vi "Main.vi"() -> ()   [LabVIEW 2014]
uses:
  Types/Lamp.ctl
  Types/TempCont.ctl
  Types/HeatingMode.ctl
  Types/Cases.ctl
  Types/DataCluster.ctl
  Types/Humans.ctl
  Types/HumanArray.ctl
  Types/Rooms.ctl
  Types/TemperatureControlData.ctl
  Types/RoomPositions.ctl
  <vilib>/Utility/miscctls.llb/LVPositionTypeDef.ctl
  Types/StartingPositions.ctl
  Types/LightCases.ctl
  Types/TemperatureArray.ctl
  Types/FVGFuncts.ctl
  <vilib>/Utility/error.llb/DialogType.ctl
  Types/MoveActions.ctl
  <vilib>/Utility/error.llb/Error Cluster From Error Code.vi
  <vilib>/Utility/file.llb/Read From Spreadsheet File (string).vi
  <vilib>/ErrorRing/Error Ring.xnode
panel:
  in  "Update Settings":bool
  out "F0 Temp Chart":dbl(graph)
  out "F1 Temp Chart":dbl(graph)
  out "Kinti hõmérséklet":dbl
  out "F1 Gain":dbl
  out "F0 Gain":dbl
  out "RIASZTÁS":bool
  out "Óra":string
  in  "Nyitott ablakok":i8 min=0 max=13 step=1
  in  "Riasztó":bool
  out "Vezérlés F1":T1
  out "Fûtési hõm. F1":dbl
  out "Aktuális hõm. F1":dbl
  in  "Kívánt hõm. F1":T2=22.0 min=10.0 max=30.0 step=0.5
  out "Vezérlés F0":T1
  out "Fûtési hõm. F0":dbl
  out "Aktuális hõm. F0":dbl
  in  "Kívánt hõm. F0":T2=22.0 min=10.0 max=30.0 step=0.5
  in  "Világítás":bool
  out "Stopped":bool
  out "EM Lámpa":T3
  out "LH Lámpa":T3
  out "EF Lámpa":T3
  out "HSZ1 Lámpa":T3
  out "HSZ2 Lámpa":T3
  out "KÉ Lámpa":T3
  out "FM Lámpa":T3
  out "FF Lámpa":T3
  out "N Lámpa":T3
  out "B Lámpa":T3
  in  "Choose Button":bool
  in  "Human 6 Button":bool
  in  "Human 5 Button":bool
  in  "Human 4 Button":bool
  in  "Human 3 Button":bool
  in  "Human 2 Button":bool
  in  "Human 1 Button":bool
  in  "Remove Button":bool
  in  "Add Button":bool
  in  "Next Button":bool
  in  "Previous Button":bool
  in  "Down Button":bool
  in  "Up Button":bool
  in  "Stop Button":bool
  in  "Human 6":u16(ring)
  in  "Human 5":u16(ring)
  in  "Human 4":u16(ring)
  in  "Human 3":u16(ring)
  in  "Human 2":u16(ring)
  in  "Human 1":u16(ring)
  # "Családtagok"
  # "Navigáció"
  # "Elsõ Emeleti Termosztát"
  # "Földszinti Termosztát"
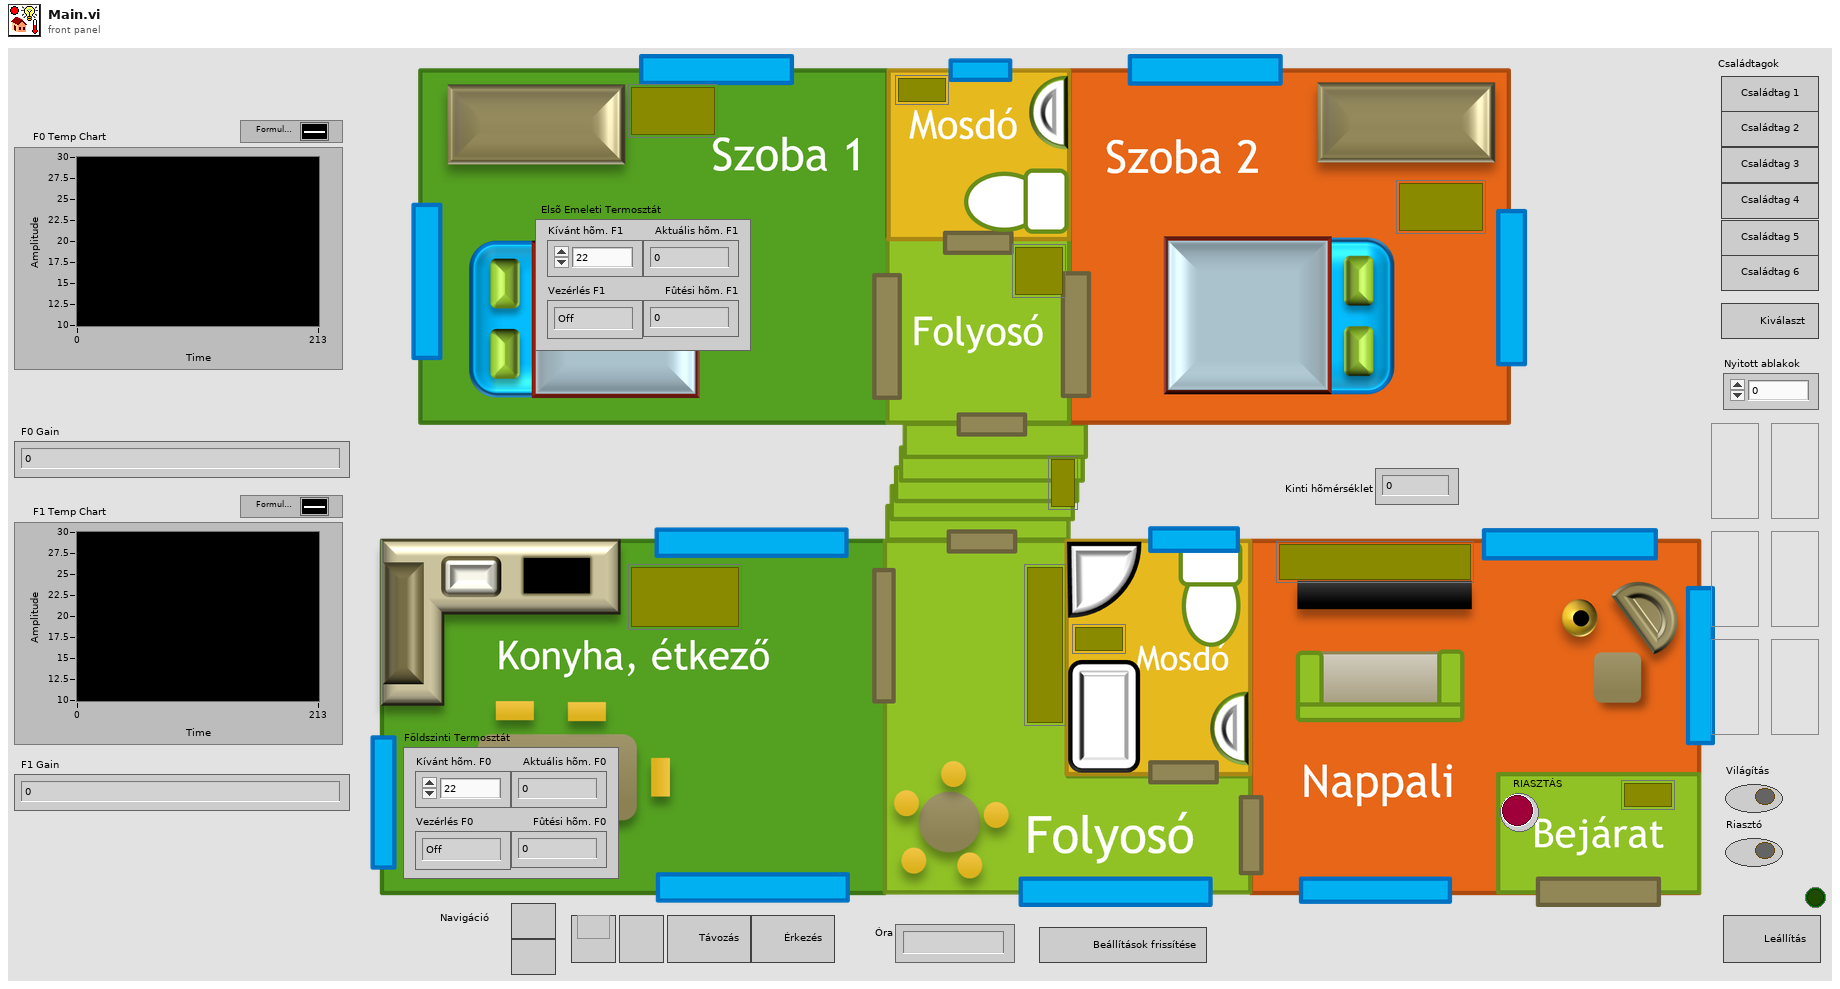
[diagram p1: front panel]
types:
  T1 = typedef "HeatingMode.ctl" = enum16{"Off", "Heating", "Cooling"}
  T2 = typedef "TempCont.ctl" = dbl
  T3 = typedef "Lamp.ctl" = bool
  T4 = typedef "LightCases.ctl" = enum16{"Start", "Update", "Stop"}
  T5 = typedef "FVGFuncts.ctl" = enum16{"Init", "Set Data", "Get Data"}
  T6 = typedef "TemperatureArray.ctl" = dbl[]
  T7 = typedef "TemperatureControlData.ctl" = cluster{"Open windows":dbl, "Floor 0 Heating":T1, "Floor 1 Heating":T1, "Heating Temp":dbl}
  T8 = typedef "HumanArray.ctl" = T9[]
  T9 = typedef "Rooms.ctl" = enum16{"Sehol", "Elõszoba", "Nappali", "Konyha", "Földszinti mosdó", "Földszinti folyosó", "Lépcsõ", "Emeleti folyosó", "Emeleti mosdó", "Hálószoba 1", "Hálószoba 2"}
  T10 = typedef "StartingPositions.ctl" = T11[]
  T11 = typedef "LVPositionTypeDef.ctl" = cluster{"Left":i32, "Top":i32}
  T12 = typedef "RoomPositions.ctl" = T11[]
  T13 = typedef "DataCluster.ctl" = cluster{"Controlled Human":T14, "Human Positions":T8, "NumOfHumans":u8, "TemperatureData":T7, "Floor0 Temp":dbl, "Floor1 Temp":dbl}
  T14 = typedef "Humans.ctl" = enum16{"No Human", "Human 1", "Human 2", "Human 3", "Human 4", "Human 5", "Human 6"}
  T15 = typedef "Cases.ctl" = enum16{"Init", "UpdateWord", "UpdateHuman", "UpdatePositions", "UpdateHeating", "UpdateTemperature", "UpdateLights", "Close", "Stop"}
  T16 = typedef "MoveActions.ctl" = enum16{"Move", "Get in", "Leave"}
  T17 = typedef "DialogType.ctl" = u16
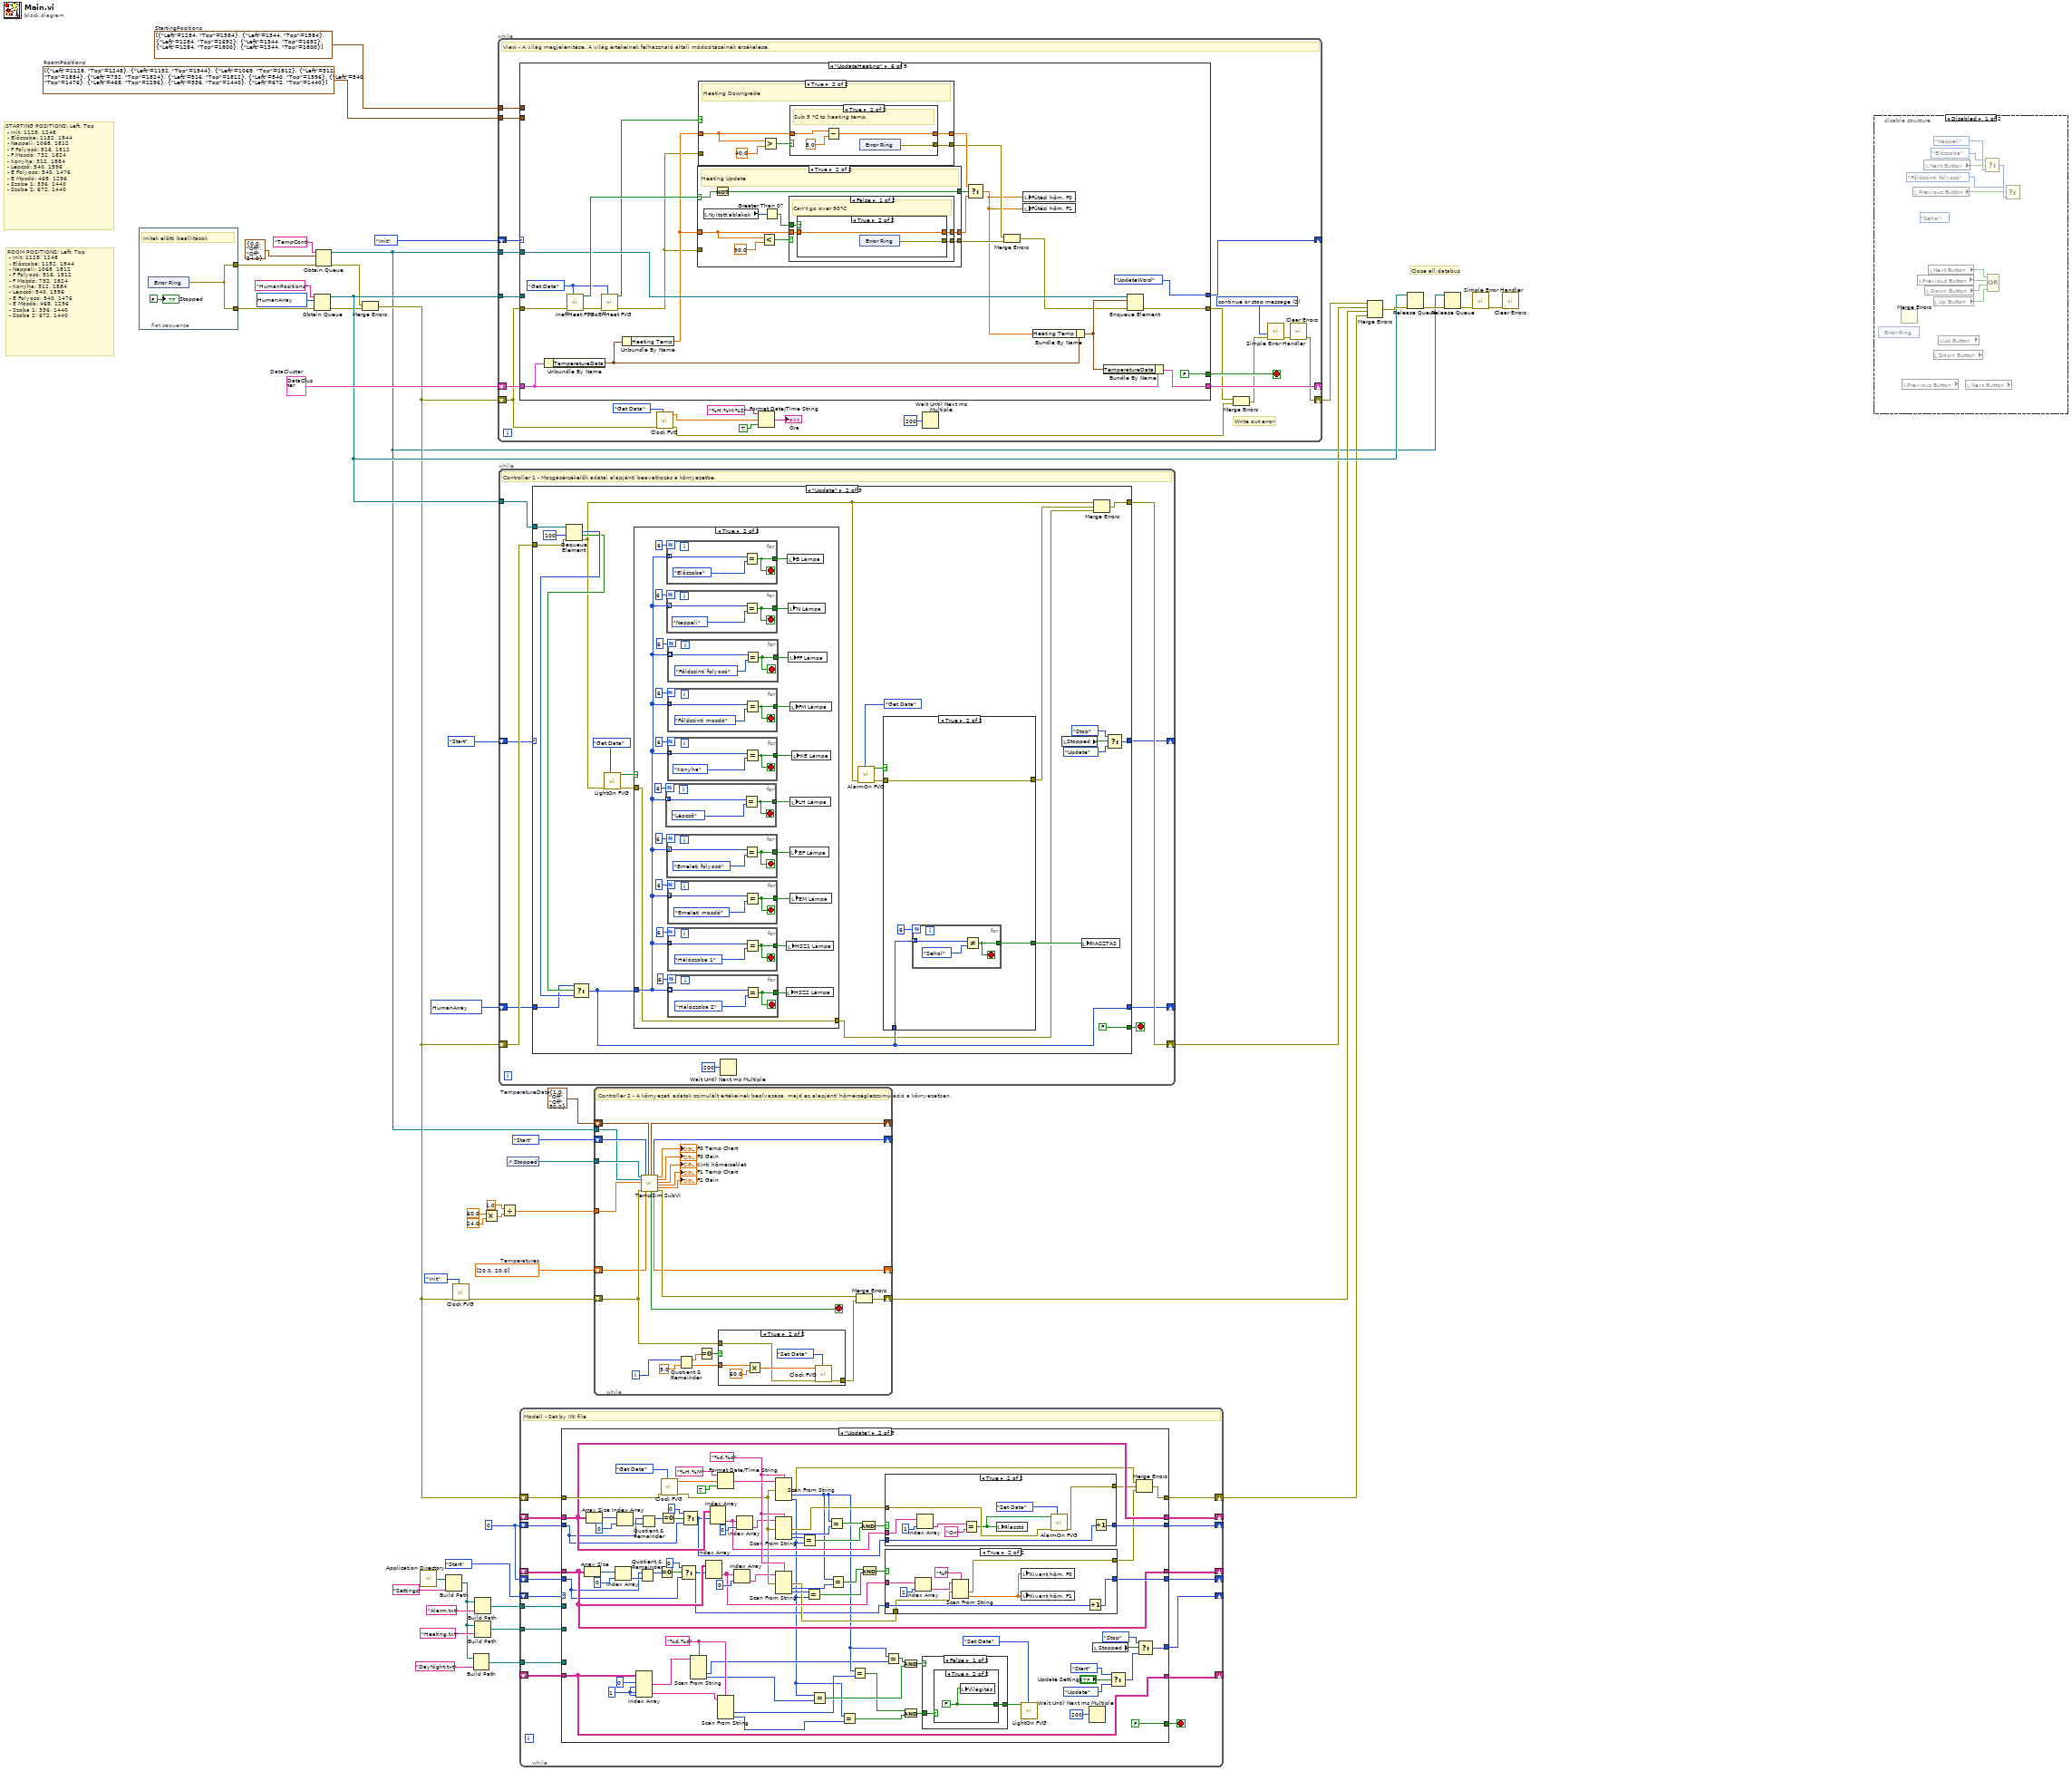
[diagram p0: block diagram]
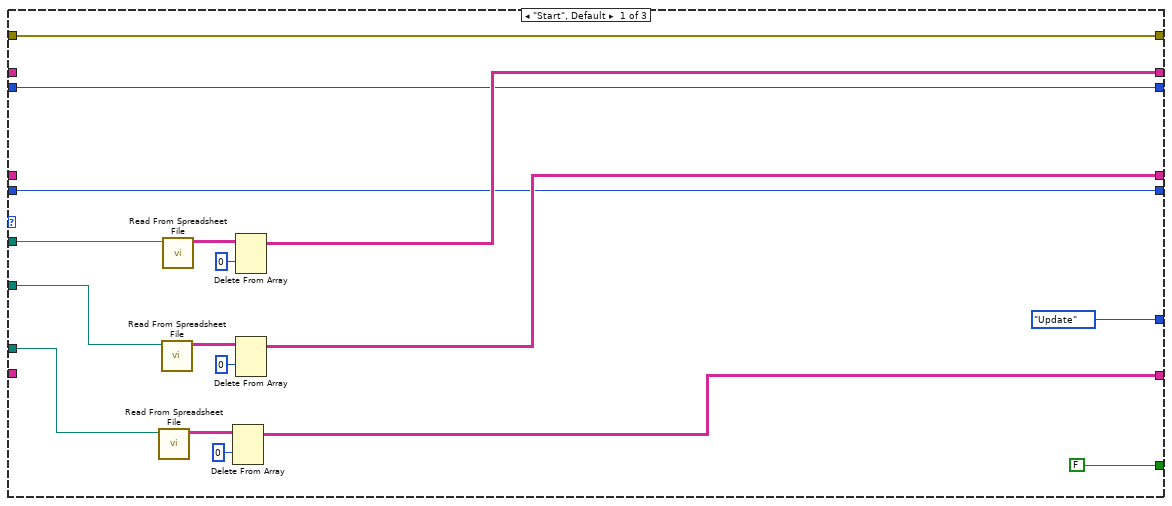
[diagram p2: hidden frame]
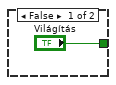
[diagram p3: hidden frame]
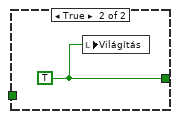
[diagram p4: hidden frame]
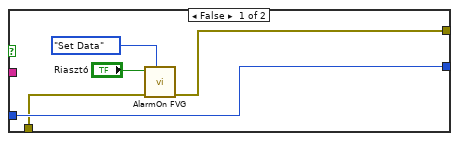
[diagram p5: hidden frame]
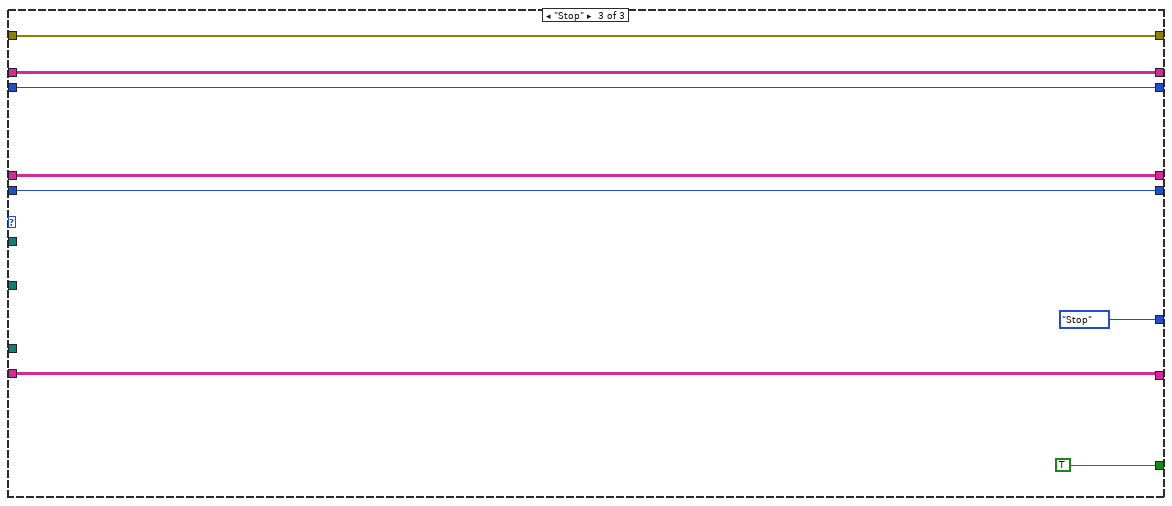
[diagram p7: hidden frame]
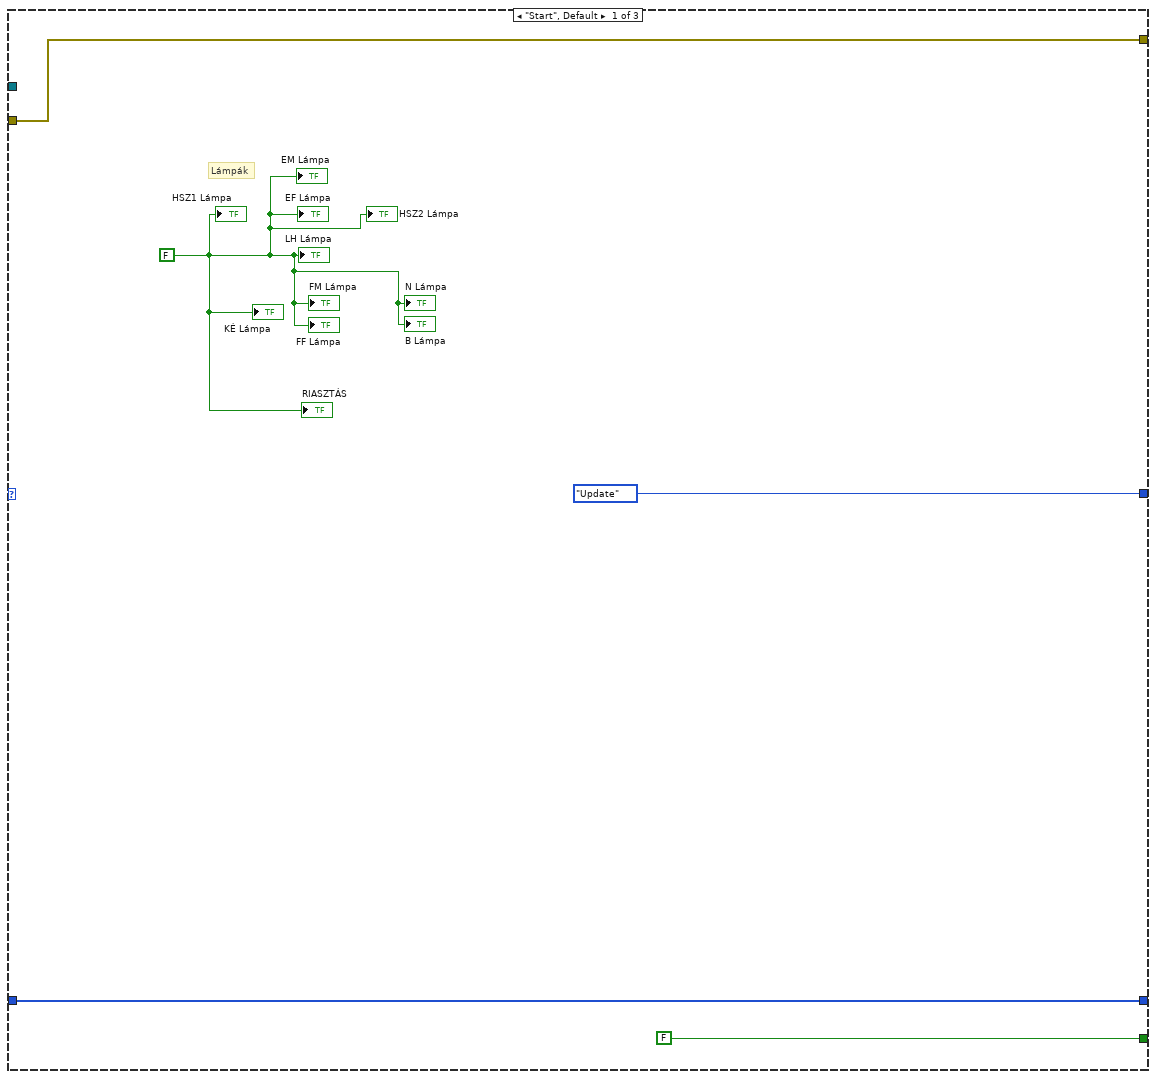
[diagram p9: hidden frame]
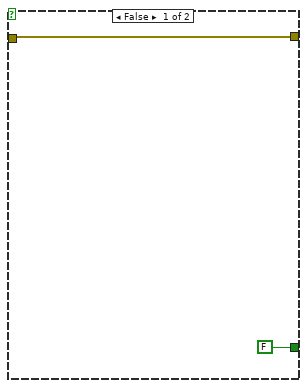
[diagram p10: hidden frame]
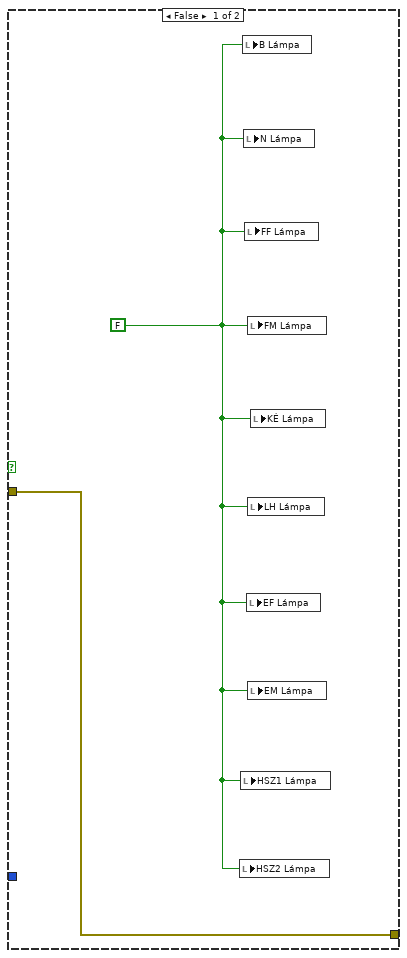
[diagram p11: hidden frame]
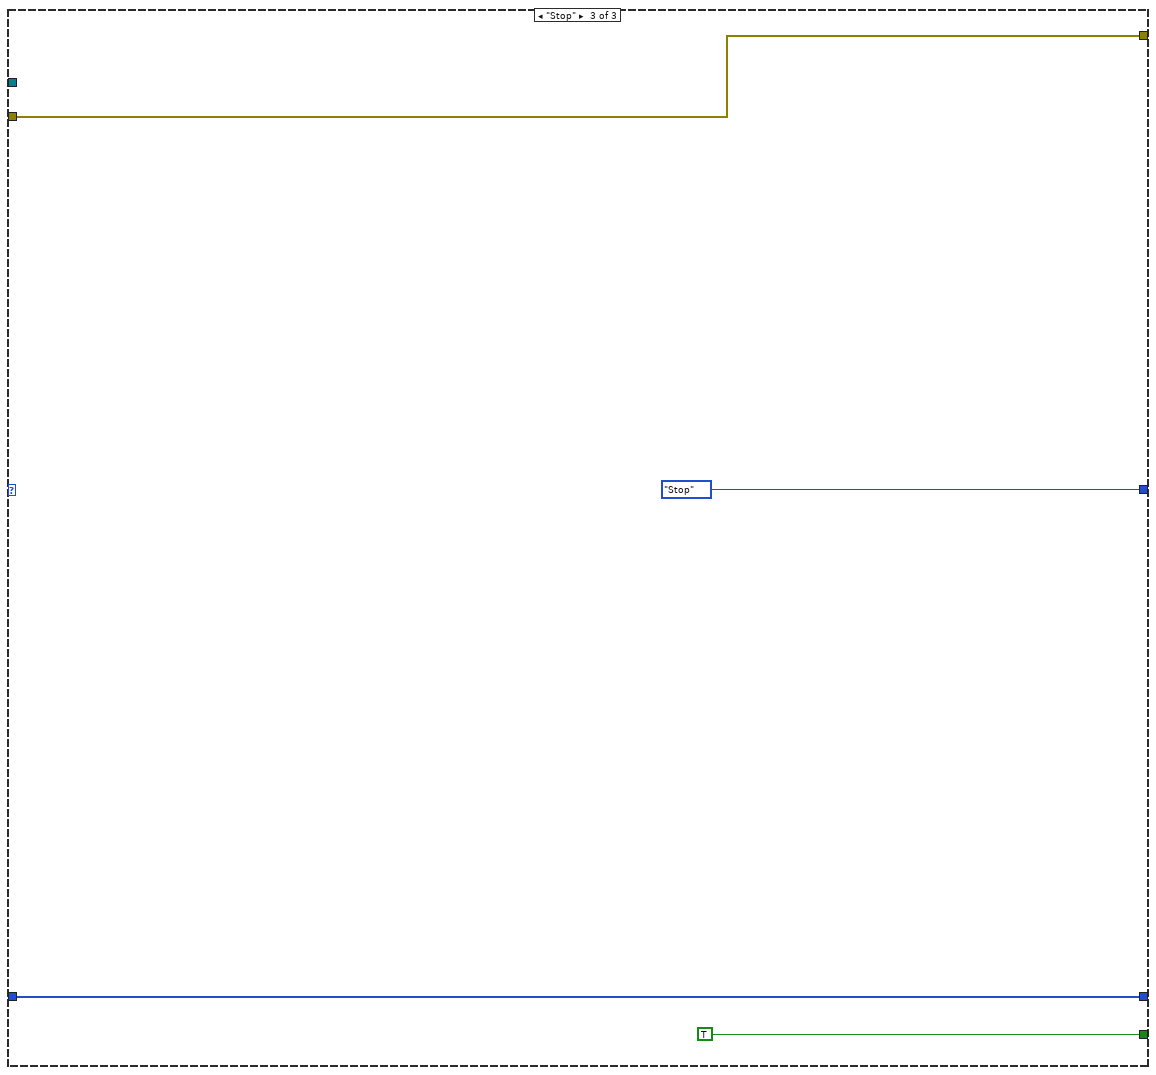
[diagram p12: hidden frame]
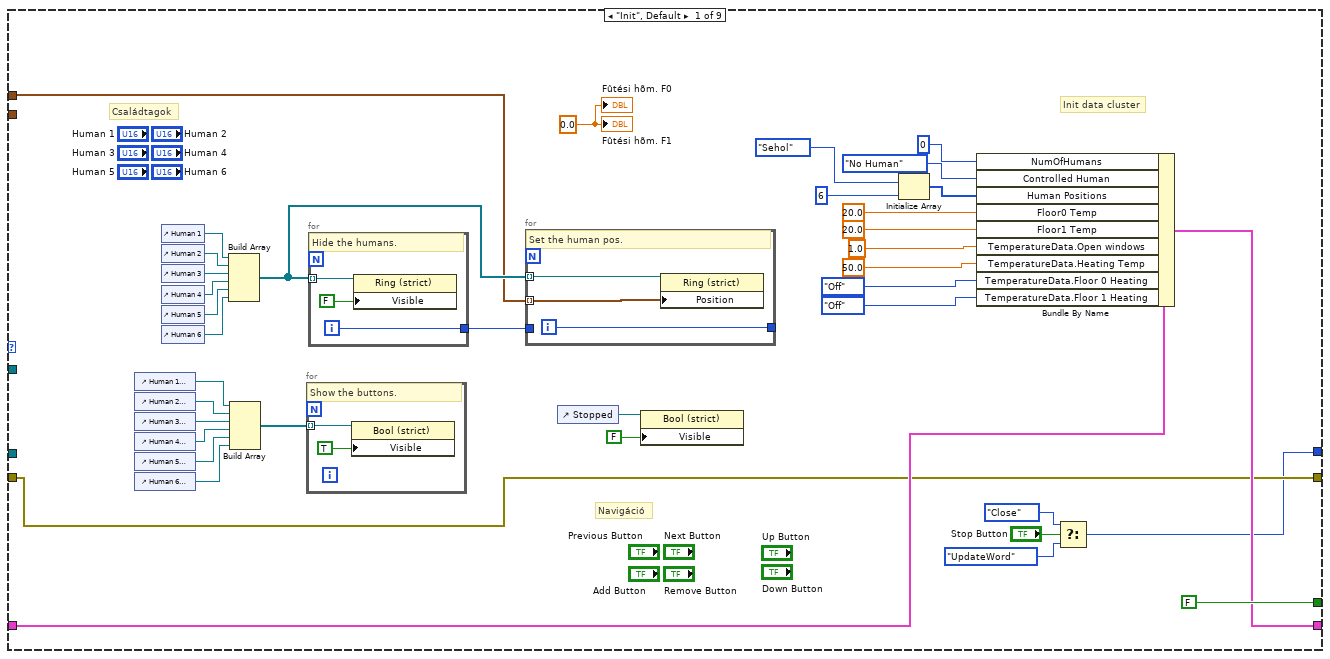
[diagram p14: hidden frame]
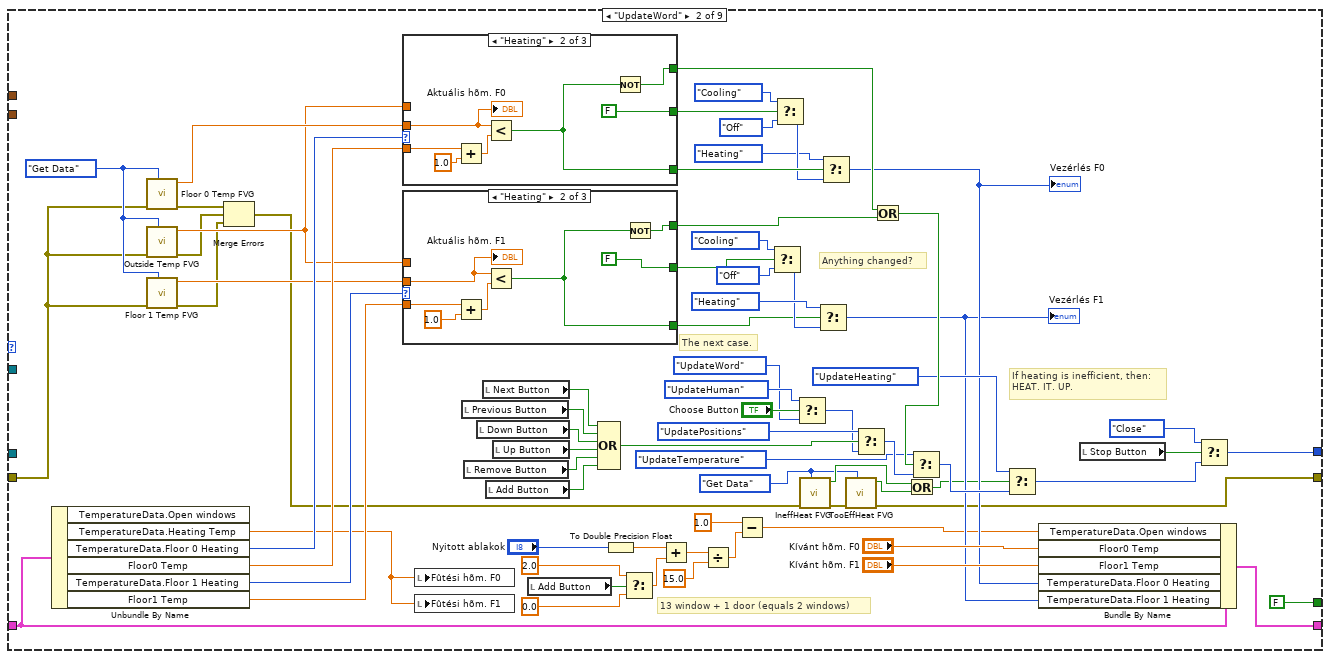
[diagram p15: hidden frame]
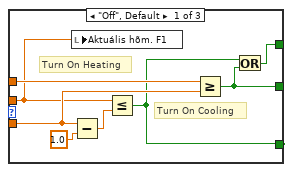
[diagram p16: hidden frame]
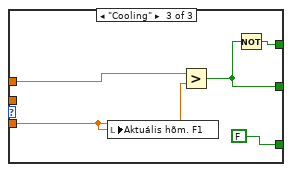
[diagram p17: hidden frame]
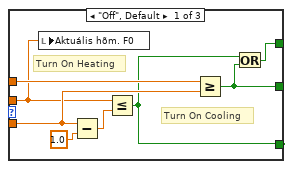
[diagram p18: hidden frame]
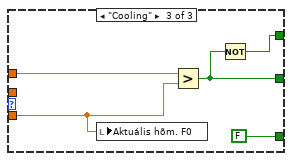
[diagram p19: hidden frame]
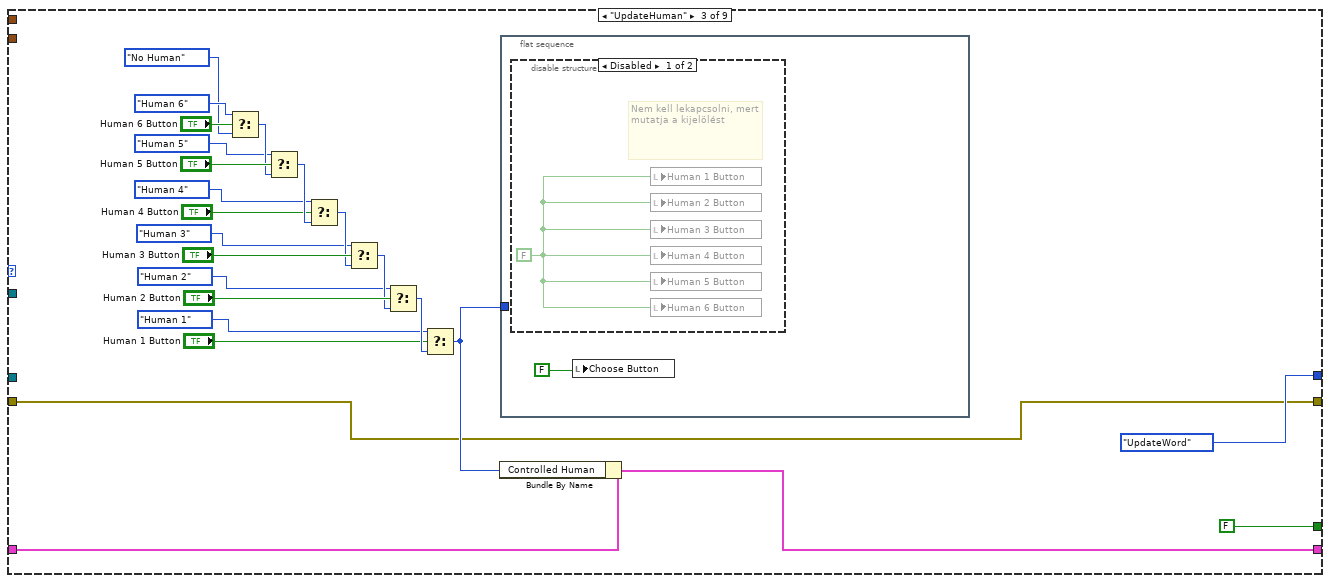
[diagram p20: hidden frame]
diagram:
  w3 = 0 ("index (row)")
  w21 = T6 [20.0, 20.0]  # Temperatures
  w22 = T7 {"Open windows"=1.0, "Floor 0 Heating"=enum."Off", "Floor 1 Heating"=enum."Off", "Heating Temp"=50.0}  # TemperatureData
  w36 = T8 [enum."Sehol", enum."Sehol", enum."Sehol", enum."Sehol", enum."Sehol", enum."Sehol", enum."Sehol", enum."Sehol", enum."Sehol", enum."Sehol", enum."Sehol", enum."Sehol"] items=["Sehol", "Elõszoba", "Nappali", "Konyha", "Földszinti mosdó", "Földszinti folyosó", "Lépcsõ", "Emeleti folyosó", "Emeleti mosdó", "Hálószoba 1", "Hálószoba 2"] ("Human Positions")
  w43 = T8 [enum."Sehol", enum."Sehol", enum."Sehol", enum."Sehol", enum."Sehol", enum."Sehol", enum."Sehol", enum."Sehol", enum."Sehol", enum."Sehol", enum."Sehol", enum."Sehol"] items=["Sehol", "Elõszoba", "Nappali", "Konyha", "Földszinti mosdó", "Földszinti folyosó", "Lépcsõ", "Emeleti folyosó", "Emeleti mosdó", "Hálószoba 1", "Hálószoba 2"] ("Human Positions")
  w44 = T10 [{"Left"=1284, "Top"=1584}, {"Left"=1344, "Top"=1584}, {"Left"=1284, "Top"=1692}, {"Left"=1344, "Top"=1692}, {"Left"=1284, "Top"=1800}, {"Left"=1344, "Top"=1800}]  # StartingPositions
  w45 = T12 [{"Left"=1128, "Top"=1248}, {"Left"=1152, "Top"=1944}, {"Left"=1068, "Top"=1812}, {"Left"=312, "Top"=1884}, {"Left"=732, "Top"=1824}, {"Left"=516, "Top"=1812}, {"Left"=540, "Top"=1596}, {"Left"=540, "Top"=1476}, {"Left"=468, "Top"=1296}, {"Left"=336, "Top"=1440}, {"Left"=672, "Top"=1440}]  # RoomPositions
  w46 = T13 {"Controlled Human"=enum."No Human", "Human Positions"=[], "NumOfHumans"=0, "TemperatureData"={"Open windows"=1.0, "Floor 0 Heating"=enum."Off", "Floor 1 Heating"=enum."Off", "Heating Temp"=50.0}, "Floor0 Temp"=24.0, "Floor1 Temp"=24.0}  # DataCluster
  # "Close all databus"
  # "STARTING POSITIONS: Left, Top\n - Init: 1128, 1248 \n - Elõszoba: 1152, 1944\n - Nappali: 1068, 1812\n - F Folyosó: 516, 1812\n - F Mosdó: 732, 1824 \n - Konyha: 312, 1884\n - Lépcsõ: 540, 1596\n - E Folyosó: 540, 1476\n - E Mosdó: 468, 1296\n - Szoba 1: 336, 1440\n - Szoba 2: 672, 1440"
  # "ROOM POSITIONS: Left, Top\n - Init: 1128, 1248 \n - Elõszoba: 1152, 1944\n - Nappali: 1068, 1812\n - F Folyosó: 516, 1812\n - F Mosdó: 732, 1824 \n - Konyha: 312, 1884\n - Lépcsõ: 540, 1596\n - E Folyosó: 540, 1476\n - E Mosdó: 468, 1296\n - Szoba 1: 336, 1440\n - Szoba 2: 672, 1440"
  n1 = flat-sequence {
    tunnel: [w48] -> w41
    tunnel: [w48] -> w35
    frame #0 {
      # "Initek elõtti beállítások"
      n2 = xnode "Error Ring"() -> ("error out"=w48:errorcluster)
      "Stopped" <- FALSE ("Stopped")
    }
  }
  n3 = Obtain Queue(name (unnamed)="HumanPositions", element data type=w43, error in (no error)=w41) -> (queue out=w39:refnum<queue>, error out=w31:errorcluster)  [unwired: 2 in, 1 out]
  n4 = Obtain Queue(name (unnamed)="TempCont", element data type=T7 {"Open windows"=0.0, "Floor 0 Heating"=enum."Off", "Floor 1 Heating"=enum."Off", "Heating Temp"=24.0} ("TemperatureData"), error in (no error)=w35) -> (queue out=w7:refnum<queue>, error out=w32:errorcluster)  [unwired: 2 in, 1 out]
  n5 = Merge Errors(w32, w31) -> (w15:errorcluster)
  n6 = call <vilib>:"Application Directory.vi"() -> ("Application Directory"=w13:path)
  n7 = Build Path(base path=w13, name or relative path="Settings") -> (appended path=w4:path)
  n8 = call "Clock FVG.vi"("Mode"=FVGFuncts."Init" ("Enum"), "Error In"=w15) -> ("Error Out"=w20:errorcluster)  [unwired: 8 in, 1 out]
  n9 = Build Path(base path=w4, name or relative path="DayNight.txt") -> (appended path=w5:path)
  n10 = Build Path(base path=w4, name or relative path="Alarm.txt") -> (appended path=w9:path)
  n11 = Build Path(base path=w4, name or relative path="Heating.txt") -> (appended path=w8:path)
  n12 = Multiply(x=60.0, y=24.0) -> (x*y=w29:dbl)
  n13 = while {
    shift-right: [w65] -> _
    shift-left: Cases."Init" -> [w72]
    shift-right: [w69] -> _
    shift-left: w46 -> [w70]
    tunnel: w45 -> [w64]
    tunnel: w44 -> [w63]
    tunnel: w39 -> [w67]
    shift-right: [w51] -> w24
    shift-left: w15 -> [w55]
    tunnel: w7 -> [w66]
    stop <- w71 stop-if-true
    w53 = T17 2 items=["no dialog", "OK message", "continue or stop message", "OK message + warnings", "continue/stop + warnings"] ("type of dialog (OK msg:1)")
    # "Write out error"
    # "View - A világ megjelenítése, A világ értékeinek felhasználó általi módositásainak érzékelése."
    n14 = case shown="\"UpdateHeating\"" w72 {
      tunnel: [FALSE FALSE FALSE FALSE FALSE FALSE FALSE FALSE TRUE] -> w71
      tunnel: [w74 w136 Cases."UpdateWord" Cases."UpdateLights" Cases."UpdateWord" Cases."UpdateWord" Cases."UpdateWord" Cases."Stop" Cases."Stop"] -> w65
      tunnel: w70 -> [w109 w154 w235 w268 w480 w501 w557 w579 w590]
      tunnel: [w105 w153 w234 w263 w480 w500 w557 w579 w590] -> w69
      tunnel: w64 -> [_ _ _ w264 _ _ _ _ _]
      tunnel: w63 -> [w88 _ _ _ _ _ _ _ _]
      tunnel: w55 -> [w86 w174 w232 w259 w478 w503 w560 w564 w589]
      tunnel: w67 -> [_ _ _ _ w479 _ _ _ _]
      tunnel: [w86 w121 w232 w258 w476 w499 w559 w564 w589] -> w59
      tunnel: w66 -> [_ _ _ _ _ w496 w558 _ _]
      frame "Init", Default {
        w73 = 0.0 ("Fûtési hõm. F1")
        # "Családtagok"
        # "Navigáció"
        # "Init data cluster"
        n15 = control-ref of="Human 1 Button"() -> (w92:refnum<vi>)
        n16 = control-ref of="Human 2 Button"() -> (w91:refnum<vi>)
        n17 = control-ref of="Human 3 Button"() -> (w96:refnum<vi>)
        n18 = control-ref of="Human 4 Button"() -> (w93:refnum<vi>)
        n19 = control-ref of="Human 5 Button"() -> (w94:refnum<vi>)
        n20 = control-ref of="Human 6 Button"() -> (w95:refnum<vi>)
        n21 = control-ref of="Human 1"() -> (w101:refnum<vi>)
        n22 = control-ref of="Human 2"() -> (w100:refnum<vi>)
        n23 = control-ref of="Human 3"() -> (w102:refnum<vi>)
        n24 = control-ref of="Human 4"() -> (w97:refnum<vi>)
        n25 = control-ref of="Human 5"() -> (w98:refnum<vi>)
        n26 = control-ref of="Human 6"() -> (w99:refnum<vi>)
        n27 = Build Array(w101, w100, w102, w97, w98, w99) -> (w89:refnum<vi>[])
        n28 = Build Array(w92, w91, w96, w93, w94, w95) -> (w90:refnum<vi>[])
        n29 = for {
          tunnel: w90 -> [w115] mode=indexing
          # "Show the buttons."
          n30 = property class="Bool (strict)"(reference=w115, "Visible"=TRUE) -> ()  [unwired: 1 in, 2 out]
        }
        n31 = for {
          tunnel: [w118] -> w87
          tunnel: w89 -> [w117] mode=indexing
          i -> [w118]
          # "Hide the humans."
          n32 = property class="Ring (strict)"(reference=w117, "Visible"=FALSE) -> ()  [unwired: 1 in, 2 out]
        }
        n33 = for {
          tunnel: [w113] -> _
          tunnel: w89 -> [w112] mode=indexing
          tunnel: w88 -> [w111] mode=indexing
          tunnel: w87 -> [_]
          i -> [w113]
          # "Set the human pos."
          n34 = property class="Ring (strict)"(reference=w112, "Position"=w111) -> ()  [unwired: 1 in, 2 out]
        }
        n35 = control-ref of="Stopped"() -> (w84:refnum<vi>)
        n36 = property class="Bool (strict)"(reference=w84, "Visible"=FALSE) -> ()  [unwired: 1 in, 2 out]
        n37 = Initialize Array(Rooms."Sehol" ("element"), 6 ("dimension size")) -> (w106:T9[])
        n38 = Bundle By Name(cluster=w109, "NumOfHumans"=u8 0, "Controlled Human"=Humans."No Human", "Human Positions"=w106, "Floor0 Temp"=20.0 ("Floor 0 Temperature"), "Floor1 Temp"=20.0 ("Floor 0 Temperature"), "TemperatureData.Open windows"=1.0 ("Floor 0 Temperature"), "TemperatureData.Heating Temp"=50.0 ("Floor 0 Temperature"), "TemperatureData.Floor 0 Heating"=HeatingMode."Off" ("Floor 0 Heating"), "TemperatureData.Floor 1 Heating"=HeatingMode."Off" ("Floor 0 Heating")) -> (w105:T13)
        n39 = Select(t=Cases."Close", s="Stop Button", f=Cases."UpdateWord") -> (s? t:f=w74:T15)
        "Fûtési hõm. F1" <- w73
        "Fûtési hõm. F0" <- w73
      }
      frame "UpdateWord" {
        w123 = FVGFuncts."Get Data" ("Mode")
        w175 = FVGFuncts."Get Data" ("Enum")
        # "13 window + 1 door (equals 2 windows)"
        # "If heating is inefficient, then: \nHEAT. IT. UP."
        # "Anything changed?"
        # "The next case."
        n40 = Unbundle By Name(w154) -> ("TemperatureData.Heating Temp"=w142:dbl, "TemperatureData.Floor 0 Heating"=w176:T1, "Floor0 Temp"=w177:dbl, "TemperatureData.Floor 1 Heating"=w172:T1, "Floor1 Temp"=w173:dbl)  [unwired: 1 out]
        n41 = call "Floor 0 Temp FVG.vi"("Mode"=w175, "Error In"=w174) -> ("Error Out"=w157:errorcluster, "Data Out"=w178:dbl)  [unwired: 8 in]
        n42 = call "Outside Temp FVG.vi"("Mode"=w175, "Error In"=w174) -> ("Error Out"=w155:errorcluster, "Data Out"=w170:dbl)  [unwired: 8 in]
        n43 = call "Floor 1 Temp FVG.vi"("Mode"=w175, "Error In"=w174) -> ("Error Out"=w156:errorcluster, "Data Out"=w171:dbl)  [unwired: 8 in]
        n44 = Merge Errors(w157, w155, w156) -> (w140:errorcluster)
        n45 = case shown="\"Heating\"" w176 {
          tunnel: w178 -> [w212 w220 _]
          tunnel: w177 -> [w217 w226 w227]
          tunnel: w170 -> [w216 _ w230]
          tunnel: [w214 w221 FALSE] -> w168
          tunnel: [w215 FALSE w229] -> w169
          tunnel: [w213 w222 w228] -> w149
          frame "Off", Default {
            # "Turn On Cooling"
            # "Turn On Heating"
            n46 = local write "Aktuális hõm. F0"(w212) -> ()
            n47 = Subtract(x=w217, y=1.0) -> (x-y=w218:dbl)
            n48 = Less Or Equal?(x=w212, y=w218) -> (x <= y?=w214:bool)
            n49 = Greater Or Equal?(x=w216, y=w217) -> (x >= y?=w215:bool)
            n50 = Or(x=w214, y=w215) -> (x .or. y?=w213:bool)
          }
          frame "Heating" {
            n51 = Add(x=w226, y=1.0) -> (x+y=w224:dbl)
            n52 = Less?(x=w220, y=w224) -> (x < y?=w221:bool)
            n53 = Not(x=w221) -> (.not. x?=w222:bool)
            "Aktuális hõm. F0" <- w220
          }
          frame "Cooling" {
            n54 = local write "Aktuális hõm. F0"(w227) -> ()
            n55 = Greater?(x=w230, y=w227) -> (0:w229:bool)
            n56 = Not(x=w229) -> (.not. x?=w228:bool)
          }
        }
        n57 = case shown="\"Heating\"" w172 {
          tunnel: w171 -> [w192 w200 _]
          tunnel: w173 -> [w197 w206 w207]
          tunnel: w170 -> [w196 _ w210]
          tunnel: [w194 w201 FALSE] -> w159
          tunnel: [w193 FALSE w209] -> w158
          tunnel: [w195 w202 w208] -> w150
          frame "Off", Default {
            # "Turn On Cooling"
            # "Turn On Heating"
            n58 = local write "Aktuális hõm. F1"(w192) -> ()
            n59 = Subtract(x=w197, y=1.0) -> (x-y=w198:dbl)
            n60 = Less Or Equal?(x=w192, y=w198) -> (x <= y?=w194:bool)
            n61 = Greater Or Equal?(x=w196, y=w197) -> (x >= y?=w193:bool)
            n62 = Or(x=w194, y=w193) -> (x .or. y?=w195:bool)
          }
          frame "Heating" {
            n63 = Add(x=w206, y=1.0) -> (x+y=w204:dbl)
            n64 = Less?(x=w200, y=w204) -> (x < y?=w201:bool)
            n65 = Not(x=w201) -> (.not. x?=w202:bool)
            "Aktuális hõm. F1" <- w200
          }
          frame "Cooling" {
            n66 = local write "Aktuális hõm. F1"(w207) -> ()
            n67 = Greater?(x=w210, y=w207) -> (0:w209:bool)
            n68 = Not(x=w209) -> (.not. x?=w208:bool)
          }
        }
        n69 = local write "Fûtési hõm. F0"(w142) -> ()
        n70 = local write "Fûtési hõm. F1"(w142) -> ()
        n71 = local read "Previous Button"() -> (w182:bool)
        n72 = local read "Remove Button"() -> (w183:bool)
        n73 = local read "Down Button"() -> (w186:bool)
        n74 = local read "Next Button"() -> (w185:bool)
        n75 = local read "Add Button"() -> (w184:bool)
        n76 = local read "Up Button"() -> (w187:bool)
        n77 = local read "Add Button"() -> (w128:bool)
        n78 = Compound Arithmetic op=OR(w185, w182, w186, w187, w183, w184) -> (w180:bool)
        n79 = To Double Precision Float(number="Nyitott ablakok") -> (double precision float=w132:dbl)
        n80 = Select(t=2.0, s=w128, f=0.0) -> (s? t:f=w131:dbl)
        n81 = Add(x=w132, y=w131) -> (x+y=w127:dbl)
        n82 = Divide(x=w127, y=15.0) -> (x/y=w125:dbl)
        n83 = Subtract(x=1.0, y=w125) -> (x-y=w135:dbl)
        n84 = Select(t=HeatingMode."Cooling" ("HeatingMode"), s=w158, f=HeatingMode."Off" ("HeatingMode")) -> (s? t:f=w160:T1)
        n85 = Select(t=HeatingMode."Cooling" ("HeatingMode"), s=w169, f=HeatingMode."Off" ("HeatingMode")) -> (s? t:f=w167:T1)
        n86 = Select(t=Cases."UpdateHuman", s="Choose Button", f=Cases."UpdateWord") -> (s? t:f=w141:T15)
        n87 = call "IneffHeat FVG.vi"("Mode"=w123, "Error In"=w140) -> ("Error Out"=w122:errorcluster, "Data Out"=w124:bool)  [unwired: 8 in]
        n88 = Select(t=HeatingMode."Heating" ("HeatingMode"), s=w159, f=w160) -> (s? t:f=w143:T1)
        "Vezérlés F1" <- w143
        n89 = Select(t=HeatingMode."Heating" ("HeatingMode"), s=w168, f=w167) -> (s? t:f=w144:T1)
        "Vezérlés F0" <- w144
        n90 = call "TooEffHeat FVG.vi"("Mode"=w123, "Error In"=w122) -> ("Error Out"=w121:errorcluster, "Data Out"=w120:bool)  [unwired: 8 in]
        n91 = Select(t=Cases."UpdatePositions", s=w180, f=w141) -> (s? t:f=w179:T15)
        n92 = Or(x=w149, y=w150) -> (x .or. y?=w148:bool)
        n93 = Or(x=w124, y=w120) -> (x .or. y?=w119:bool)
        n94 = Select(t=Cases."UpdateTemperature", s=w148, f=w179) -> (s? t:f=w146:T15)
        n95 = Select(t=Cases."UpdateHeating", s=w119, f=w146) -> (s? t:f=w137:T15)
        n96 = Bundle By Name(cluster=w154, "TemperatureData.Open windows"=w135, "Floor0 Temp"="Kívánt hõm. F0", "Floor1 Temp"="Kívánt hõm. F1", "TemperatureData.Floor 0 Heating"=w144, "TemperatureData.Floor 1 Heating"=w143) -> (w153:T13)
        n97 = local read "Stop Button"() -> (w139:bool)
        n98 = Select(t=Cases."Close", s=w139, f=w137) -> (s? t:f=w136:T15)
      }
      frame "UpdateHuman" {
        n99 = Select(t=Humans."Human 6", s="Human 6 Button", f=Humans."No Human") -> (s? t:f=w251:T14)
        n100 = Select(t=Humans."Human 5", s="Human 5 Button", f=w251) -> (s? t:f=w248:T14)
        n101 = Select(t=Humans."Human 4", s="Human 4 Button", f=w248) -> (s? t:f=w245:T14)
        n102 = Select(t=Humans."Human 3", s="Human 3 Button", f=w245) -> (s? t:f=w243:T14)
        n103 = Select(t=Humans."Human 2", s="Human 2 Button", f=w243) -> (s? t:f=w242:T14)
        n104 = Select(t=Humans."Human 1", s="Human 1 Button", f=w242) -> (s? t:f=w233:T14)
        n105 = Bundle By Name(cluster=w235, "Controlled Human"=w233) -> (w234:T13)
        n106 = flat-sequence {
          tunnel: w233 -> [_]
          frame #0 {
            n107 = disable-structure shown="Disabled" {
              frame Disabled {
                w257 = FALSE
                # "Nem kell lekapcsolni, mert mutatja a kijelölést"
                n108 = local write "Human 1 Button"(w257) -> ()
                n109 = local write "Human 2 Button"(w257) -> ()
                n110 = local write "Human 3 Button"(w257) -> ()
                n111 = local write "Human 4 Button"(w257) -> ()
                n112 = local write "Human 5 Button"(w257) -> ()
                n113 = local write "Human 6 Button"(w257) -> ()
              }
              frame Enabled {
              }
            }
            n114 = local write "Choose Button"(FALSE) -> ()
          }
        }
      }
      frame "UpdatePositions" {
        # "Choose the moving type. \n(Works if only 1 can be true)"
        n115 = local read "Remove Button"() -> (w272:bool)
        n116 = local read "Add Button"() -> (w271:bool)
        n117 = Unbundle By Name(w268) -> ("Human Positions"=w274:T8, "Controlled Human"=w276:T14, "NumOfHumans"=w265:u8)
        n118 = Select(t=MoveActions."Get in", s=w271, f=MoveActions."Move") -> (s? t:f=w261:T16)
        n119 = Select(t=MoveActions."Leave", s=w272, f=w261) -> (s? t:f=w269:T16)
        n120 = case shown="\"Get in\"" w269 {
          tunnel: w276 -> [w287 w383 w430]
          tunnel: w274 -> [w283 w386 w440]
          tunnel: [w282 w385 w438] -> w267
          tunnel: [w281 w392 w431] -> w266
          tunnel: w265 -> [w281 w393 w432]
          tunnel: w264 -> [w280 w384 w439]
          tunnel: [w279 w391 w437] -> w258
          tunnel: w259 -> [w278 w381 w428]
          frame "Move", Default {
            # "Who moves?"
            # "Where it can move?"
            n121 = Decrement(x=w287) -> (x-1=w284:T14)
            n122 = Index Array(array=w283, index=w284) -> (element=w286:T9)
            n123 = case shown="\"Sehol\", Default" w286 {
              tunnel: [Rooms."Sehol" ("element") w291 w295 w302 w306 w310 w323 w330 w343 w347 w351] -> w285
              frame "Sehol", Default {
              }
              frame "Elõszoba" {
                n124 = local read "Previous Button"() -> (w294:bool)
                n125 = Select(t=Rooms."Nappali" ("element"), s=w294, f=Rooms."Elõszoba" ("element")) -> (s? t:f=w291:T9)
              }
              frame "Nappali" {
                n126 = local read "Previous Button"() -> (w299:bool)
                n127 = local read "Next Button"() -> (w301:bool)
                n128 = Select(t=Rooms."Elõszoba" ("element"), s=w301, f=Rooms."Nappali" ("element")) -> (s? t:f=w296:T9)
                n129 = Select(t=Rooms."Földszinti folyosó" ("element"), s=w299, f=w296) -> (s? t:f=w295:T9)
              }
              frame "Konyha" {
                n130 = local read "Next Button"() -> (w305:bool)
                n131 = Select(t=Rooms."Földszinti folyosó" ("element"), s=w305, f=Rooms."Konyha" ("element")) -> (s? t:f=w302:T9)
              }
              frame "Földszinti mosdó" {
                n132 = local read "Down Button"() -> (w309:bool)
                n133 = Select(t=Rooms."Földszinti folyosó" ("element"), s=w309, f=Rooms."Földszinti mosdó" ("element")) -> (s? t:f=w306:T9)
              }
              frame "Földszinti folyosó" {
                n134 = local read "Previous Button"() -> (w320:bool)
                n135 = local read "Down Button"() -> (w319:bool)
                n136 = local read "Next Button"() -> (w322:bool)
                n137 = local read "Up Button"() -> (w318:bool)
                n138 = Select(t=Rooms."Nappali" ("element"), s=w322, f=Rooms."Földszinti folyosó" ("element")) -> (s? t:f=w317:T9)
                n139 = Select(t=Rooms."Konyha" ("element"), s=w320, f=w317) -> (s? t:f=w315:T9)
                n140 = Select(t=Rooms."Földszinti mosdó" ("element"), s=w319, f=w315) -> (s? t:f=w312:T9)
                n141 = Select(t=Rooms."Lépcsõ" ("element"), s=w318, f=w312) -> (s? t:f=w310:T9)
              }
              frame "Lépcsõ" {
                n142 = local read "Down Button"() -> (w327:bool)
                n143 = local read "Up Button"() -> (w329:bool)
                n144 = Select(t=Rooms."Emeleti folyosó" ("element"), s=w329, f=Rooms."Lépcsõ" ("element")) -> (s? t:f=w324:T9)
                n145 = Select(t=Rooms."Földszinti folyosó" ("element"), s=w327, f=w324) -> (s? t:f=w323:T9)
              }
              frame "Emeleti folyosó" {
                n146 = local read "Previous Button"() -> (w340:bool)
                n147 = local read "Down Button"() -> (w339:bool)
                n148 = local read "Next Button"() -> (w342:bool)
                n149 = local read "Up Button"() -> (w338:bool)
                n150 = Select(t=Rooms."Hálószoba 2" ("element"), s=w342, f=Rooms."Emeleti folyosó" ("element")) -> (s? t:f=w337:T9)
                n151 = Select(t=Rooms."Hálószoba 1" ("element"), s=w340, f=w337) -> (s? t:f=w335:T9)
                n152 = Select(t=Rooms."Lépcsõ" ("element"), s=w339, f=w335) -> (s? t:f=w332:T9)
                n153 = Select(t=Rooms."Emeleti mosdó" ("element"), s=w338, f=w332) -> (s? t:f=w330:T9)
              }
              frame "Emeleti mosdó" {
                n154 = local read "Down Button"() -> (w346:bool)
                n155 = Select(t=Rooms."Emeleti folyosó" ("element"), s=w346, f=Rooms."Emeleti mosdó" ("element")) -> (s? t:f=w343:T9)
              }
              frame "Hálószoba 1" {
                n156 = local read "Next Button"() -> (w350:bool)
                n157 = Select(t=Rooms."Emeleti folyosó" ("element"), s=w350, f=Rooms."Hálószoba 1" ("element")) -> (s? t:f=w347:T9)
              }
              frame "Hálószoba 2" {
                n158 = local read "Previous Button"() -> (w354:bool)
                n159 = Select(t=Rooms."Emeleti folyosó" ("element"), s=w354, f=Rooms."Hálószoba 2" ("element")) -> (s? t:f=w351:T9)
              }
            }
            n160 = case shown="\"Human 4\"" w287 {
              tunnel: [FALSE TRUE TRUE TRUE TRUE TRUE TRUE] -> w289
              tunnel: [refnum<vi> refnum ("Human 6") w370 w372 w374 w376 w377 w380] -> w288
              frame "No Human", Default {
              }
              frame "Human 1" {
                n161 = control-ref of="Human 1"() -> (w370:refnum<vi>)
              }
              frame "Human 2" {
                n162 = control-ref of="Human 2"() -> (w372:refnum<vi>)
              }
              frame "Human 3" {
                n163 = control-ref of="Human 3"() -> (w374:refnum<vi>)
              }
              frame "Human 4" {
                n164 = control-ref of="Human 4"() -> (w376:refnum<vi>)
              }
              frame "Human 5" {
                n165 = control-ref of="Human 5"() -> (w377:refnum<vi>)
              }
              frame "Human 6" {
                n166 = control-ref of="Human 6"() -> (w380:refnum<vi>)
              }
            }
            n167 = case shown="True" w289 {
              tunnel: w288 -> [_ w366]
              tunnel: w285 -> [_ w362]
              tunnel: w284 -> [_ w365]
              tunnel: w283 -> [w356 w364]
              tunnel: [w356 w360] -> w282
              tunnel: w280 -> [_ w363]
              tunnel: [w355 w359] -> w279
              tunnel: w278 -> [_ w358]
              frame False {
                n168 = xnode "Error Ring"() -> ("error out"=w355:errorcluster)
              }
              frame True {
                # "Update the position of human."
                n169 = Index Array(array=w363, index=w362) -> (element=w361:T11)
                n170 = Replace Array Subset(array=w364, new element=w362, index=w365) -> (w360:T8)
                n171 = property class="Ring (strict)"(reference=w366, error in=w358, "Position"=w361) -> (error out=w359:errorcluster)  [unwired: 1 out]
              }
            }
          }
          frame "Get in" {
            w388 = Rooms."Elõszoba" ("element")
            # "Update the position of human."
            # "Who moves?"
            n172 = Increment(x=w393) -> (x+1=w392:u8)
            n173 = Decrement(x=w383) -> (x-1=w382:T14)
            n174 = case shown="\"Human 1\"" w383 {
              tunnel: [FALSE TRUE TRUE TRUE TRUE TRUE TRUE] -> w390
              tunnel: [refnum<vi> refnum ("Human 6") w399 w402 w405 w408 w410 w414] -> w389
              tunnel: [refnum<vi> refnum ("Human 6 Button") w397 w400 w403 w406 w409 w412] -> w387
              frame "No Human", Default {
              }
              frame "Human 1" {
                n175 = control-ref of="Human 1"() -> (w399:refnum<vi>)
                n176 = control-ref of="Human 1 Button"() -> (w397:refnum<vi>)
              }
              frame "Human 2" {
                n177 = control-ref of="Human 2"() -> (w402:refnum<vi>)
                n178 = control-ref of="Human 2 Button"() -> (w400:refnum<vi>)
              }
              frame "Human 3" {
                n179 = control-ref of="Human 3"() -> (w405:refnum<vi>)
                n180 = control-ref of="Human 3 Button"() -> (w403:refnum<vi>)
              }
              frame "Human 4" {
                n181 = control-ref of="Human 4"() -> (w408:refnum<vi>)
                n182 = control-ref of="Human 4 Button"() -> (w406:refnum<vi>)
              }
              frame "Human 5" {
                n183 = control-ref of="Human 5"() -> (w410:refnum<vi>)
                n184 = control-ref of="Human 5 Button"() -> (w409:refnum<vi>)
              }
              frame "Human 6" {
                n185 = control-ref of="Human 6"() -> (w414:refnum<vi>)
                n186 = control-ref of="Human 6 Button"() -> (w412:refnum<vi>)
              }
            }
            n187 = Replace Array Subset(array=w386, new element=w388, index=w382) -> (w385:T8)
            n188 = case shown="True" w390 {
              tunnel: w389 -> [_ w424]
              tunnel: w388 -> [_ w426]
              tunnel: w384 -> [_ w425]
              tunnel: w387 -> [_ w423]
              tunnel: [w415 w418] -> w391
              tunnel: w381 -> [_ w417]
              frame False {
                n189 = xnode "Error Ring"() -> ("error out"=w415:errorcluster)
              }
              frame True {
                w422 = TRUE
                n190 = Index Array(array=w425, index=w426) -> (element=w427:T11)
                n191 = property class="Ring (strict)"(reference=w424, error in=w417, "Visible"=w422) -> (error out=w420:errorcluster)  [unwired: 1 out]
                n192 = property class="Ring (strict)"(reference=w424, error in=w417, "Position"=w427) -> (error out=w421:errorcluster)  [unwired: 1 out]
                n193 = property class="Bool (strict)"(reference=w423, error in=w417, "Visible"=w422) -> (error out=w419:errorcluster)  [unwired: 1 out]
                n194 = Merge Errors(w419, w420, w421) -> (w418:errorcluster)
              }
            }
          }
          frame "Leave" {
            w436 = Rooms."Sehol" ("element")
            # "Who moves?"
            # "Update the position of human."
            n195 = Decrement(x=w432) -> (x-1=w431:u8)
            n196 = Decrement(x=w430) -> (x-1=w429:T14)
            n197 = case shown="\"Human 1\"" w430 {
              tunnel: [FALSE TRUE TRUE TRUE TRUE TRUE TRUE] -> w434
              tunnel: [refnum<vi> refnum ("Human 6") w446 w449 w452 w455 w457 w461] -> w435
              tunnel: [refnum<vi> refnum ("Human 6 Button") w444 w447 w450 w453 w456 w459] -> w433
              frame "No Human", Default {
              }
              frame "Human 1" {
                n198 = control-ref of="Human 1"() -> (w446:refnum<vi>)
                n199 = control-ref of="Human 1 Button"() -> (w444:refnum<vi>)
              }
              frame "Human 2" {
                n200 = control-ref of="Human 2"() -> (w449:refnum<vi>)
                n201 = control-ref of="Human 2 Button"() -> (w447:refnum<vi>)
              }
              frame "Human 3" {
                n202 = control-ref of="Human 3"() -> (w452:refnum<vi>)
                n203 = control-ref of="Human 3 Button"() -> (w450:refnum<vi>)
              }
              frame "Human 4" {
                n204 = control-ref of="Human 4"() -> (w455:refnum<vi>)
                n205 = control-ref of="Human 4 Button"() -> (w453:refnum<vi>)
              }
              frame "Human 5" {
                n206 = control-ref of="Human 5"() -> (w457:refnum<vi>)
                n207 = control-ref of="Human 5 Button"() -> (w456:refnum<vi>)
              }
              frame "Human 6" {
                n208 = control-ref of="Human 6"() -> (w461:refnum<vi>)
                n209 = control-ref of="Human 6 Button"() -> (w459:refnum<vi>)
              }
            }
            n210 = Replace Array Subset(array=w440, new element=w436, index=w429) -> (w438:T8)
            n211 = case shown="True" w434 {
              tunnel: w436 -> [_ w474]
              tunnel: w439 -> [_ w473]
              tunnel: w435 -> [_ w471]
              tunnel: w433 -> [_ w470]
              tunnel: [w462 w468] -> w437
              tunnel: w428 -> [_ w464]
              frame False {
                n212 = xnode "Error Ring"() -> ("error out"=w462:errorcluster)
              }
              frame True {
                n213 = Index Array(array=w473, index=w474) -> (element=w475:T11)
                n214 = property class="Ring (strict)"(reference=w471, error in=w464, "Visible"=FALSE) -> (error out=w466:errorcluster)  [unwired: 1 out]
                n215 = property class="Bool (strict)"(reference=w470, error in=w464, "Visible"=TRUE) -> (error out=w469:errorcluster)  [unwired: 1 out]
                n216 = property class="Ring (strict)"(reference=w471, error in=w464, "Position"=w475) -> (error out=w467:errorcluster)  [unwired: 1 out]
                n217 = Merge Errors(w469, w466, w467) -> (w468:errorcluster)
              }
            }
          }
        }
        n218 = Bundle By Name(cluster=w268, "Human Positions"=w267, "NumOfHumans"=w266) -> (w263:T13)
        n219 = flat-sequence {
          tunnel: w258 -> [_]
          tunnel: w263 -> [_]
          frame #0 {
            w277 = FALSE
            n220 = local write "Next Button"(w277) -> ()
            n221 = local write "Up Button"(w277) -> ()
            n222 = local write "Down Button"(w277) -> ()
            n223 = local write "Add Button"(w277) -> ()
            n224 = local write "Previous Button"(w277) -> ()
            n225 = local write "Remove Button"(w277) -> ()
          }
        }
      }
      frame "UpdateLights" {
        n226 = Unbundle By Name(w480) -> ("Human Positions"=w477:T8)
        n227 = Enqueue Element(queue=w479, element=w477, error in (no error)=w478) -> (error out=w476:errorcluster)  [unwired: 1 in, 2 out]
      }
      frame "UpdateHeating" {
        w484 = FVGFuncts."Get Data" ("Mode")
        n228 = Unbundle By Name(w501) -> ("TemperatureData"=w498:T7)
        n229 = call "IneffHeat FVG.vi"("Mode"=w484, "Error In"=w503) -> ("Error Out"=w486:errorcluster, "Data Out"=w502:bool)  [unwired: 8 in]
        n230 = call "TooEffHeat FVG.vi"("Mode"=w484, "Error In"=w486) -> ("Error Out"=w485:errorcluster, "Data Out"=w483:bool)  [unwired: 8 in]
        n231 = Unbundle By Name(w498) -> ("Heating Temp"=w495:dbl)
        n232 = case shown="True" w502 {
          selector: w502 -> [w526 w531]
          tunnel: [w524 w534] -> w492
          tunnel: [w527 w533] -> w491
          tunnel: w485 -> [w527 _]
          tunnel: w495 -> [w524 w532]
          tunnel: [w525 w530] -> w494
          frame False {
            # "Keep heating temp., if unneded."
            n233 = Not(x=w526) -> (.not. x?=w525:bool)
          }
          frame True {
            # "Heating Update"
            n234 = local read "Nyitott ablakok"() -> (w529:i8)
            n235 = Not(x=w531) -> (.not. x?=w530:bool)
            n236 = Less?(x=w532, y=90.0) -> (x < y?=w535:bool)
            n237 = Greater Than 0?(x=w529) -> (x > 0?=w528:bool)
            n238 = case shown="False" w535 {
              tunnel: w532 -> [w540 w554]
              tunnel: [w539 w552] -> w534
              tunnel: [w537 w551] -> w533
              tunnel: w528 -> [w538 _]
              frame False {
                # "Can't go over 90°C"
                n239 = case shown="True" w538 {
                  tunnel: w540 -> [w541 w549]
                  tunnel: [w541 w549] -> w539
                  tunnel: [w542 w548] -> w537
                  frame False {
                    n240 = xnode "Error Ring"() -> ("error out"=w542:errorcluster)
                  }
                  frame True {
                    n241 = xnode "Error Ring"() -> ("error out"=w548:errorcluster)
                  }
                }
              }
              frame True {
                # "Add 5 °C to heating temp."
                n242 = Add(x=w554, y=5.0) -> (x+y=w552:dbl)
                n243 = xnode "Error Ring"() -> ("error out"=w551:errorcluster)
              }
            }
          }
        }
        n244 = case shown="True" w483 {
          tunnel: [w505 w509] -> w493
          tunnel: [w506 w508] -> w490
          tunnel: w485 -> [w506 _]
          tunnel: w495 -> [w505 w507]
          frame False {
            # "Keep heating temp., if unneded."
          }
          frame True {
            # "Heating Downgrade"
            n245 = Greater?(x=w507, y=40.0) -> (0:w510:bool)
            n246 = case shown="True" w510 {
              tunnel: w507 -> [w513 w522]
              tunnel: [w513 w520] -> w509
              tunnel: [w512 w519] -> w508
              frame False {
                # "Don't go below 40 °C"
                n247 = xnode "Error Ring"() -> ("error out"=w512:errorcluster)
              }
              frame True {
                # "Sub 5 °C to heating temp."
                n248 = Subtract(x=w522, y=5.0) -> (x-y=w520:dbl)
                n249 = xnode "Error Ring"() -> ("error out"=w519:errorcluster)
              }
            }
          }
        }
        n250 = Select(t=w493, s=w494, f=w492) -> (s? t:f=w489:dbl)
        n251 = Merge Errors(w490, w491) -> (w488:errorcluster)
        n252 = local write "Fûtési hõm. F0"(w489) -> ()
        n253 = local write "Fûtési hõm. F1"(w489) -> ()
        n254 = Bundle By Name(cluster=w498, "Heating Temp"=w489) -> (w497:T7)
        n255 = Bundle By Name(cluster=w501, "TemperatureData"=w497) -> (w500:T13)
        n256 = Enqueue Element(queue=w496, element=w497, error in (no error)=w488) -> (error out=w499:errorcluster)  [unwired: 1 in, 2 out]
      }
      frame "UpdateTemperature" {
        n257 = Unbundle By Name(w557) -> ("TemperatureData"=w556:T7)  [unwired: 2 out]
        n258 = Enqueue Element(queue=w558, element=w556, error in (no error)=w560) -> (error out=w559:errorcluster)  [unwired: 1 in, 2 out]
      }
      frame "Close" {
        # "Make them visible again"
        n259 = control-ref of="Human 1 Button"() -> (w568:refnum<vi>)
        n260 = control-ref of="Human 2 Button"() -> (w567:refnum<vi>)
        n261 = control-ref of="Human 3 Button"() -> (w572:refnum<vi>)
        n262 = control-ref of="Human 4 Button"() -> (w569:refnum<vi>)
        n263 = control-ref of="Human 5 Button"() -> (w570:refnum<vi>)
        n264 = control-ref of="Human 6 Button"() -> (w571:refnum<vi>)
        n265 = control-ref of="Stopped"() -> (w563:refnum<vi>)
        n266 = control-ref of="Human 1"() -> (w577:refnum<vi>)
        n267 = control-ref of="Human 2"() -> (w576:refnum<vi>)
        n268 = control-ref of="Human 3"() -> (w578:refnum<vi>)
        n269 = control-ref of="Human 4"() -> (w573:refnum<vi>)
        n270 = control-ref of="Human 5"() -> (w574:refnum<vi>)
        n271 = control-ref of="Human 6"() -> (w575:refnum<vi>)
        n272 = Build Array(w577, w576, w578, w573, w574, w575) -> (w565:refnum<vi>[])
        n273 = Build Array(w568, w567, w572, w569, w570, w571, w563) -> (w566:refnum<vi>[])
        n274 = for {
          tunnel: w566 -> [w583] mode=indexing
          # "Hide the buttons."
          n275 = property class="Bool (strict)"(reference=w583, "Visible"=TRUE) -> ()  [unwired: 1 in, 2 out]
        }
        n276 = for {
          tunnel: [w586] -> _
          tunnel: w565 -> [w585] mode=indexing
          i -> [w586]
          # "Hide the humans."
          n277 = property class="Ring (strict)"(reference=w585, "Visible"=TRUE) -> ()  [unwired: 1 in, 2 out]
        }
      }
      frame "Stop" {
        n278 = local write "Stopped"(TRUE ("Stopped")) -> ()
        n279 = local write "Stop Button"(FALSE ("Stop Button")) -> ()
      }
    }
    n280 = call "Clock FVG.vi"("Mode"=FVGFuncts."Get Data", "Error In"=w55) -> ("Error Out"=w54:errorcluster, "Data Out"=w56:dbl)  [unwired: 8 in]
    n281 = Format Date/Time String(time format string (%c)="%H:%M:%S", seconds (now)=w56, UTC format=TRUE) -> (date/time string=→"Óra":string)
    n282 = Wait Until Next ms Multiple(millisecond multiple=u32 200) -> ()  [unwired: 1 out]
    n283 = Merge Errors(w59, w54) -> (w58:errorcluster)
    n284 = call <vilib>:"Simple Error Handler.vi"("type of dialog (OK msg:1)"=w53, "error in (no error)"=w58) -> ("error out"=w52:errorcluster)  [unwired: 3 in, 4 out]
    n285 = call <vilib>:"Clear Errors.vi"("error in (no error)"=w52) -> ("error out"=w51:errorcluster)  [unwired: 5 in, 1 out]
  }
  n286 = while {
    tunnel: w39 -> [w601]
    shift-right: [w598] -> _
    shift-left: LightCases."Start" -> [w596]
    shift-right: [w594] -> _
    shift-left: w36 -> [w595]
    shift-right: [w599] -> w38
    shift-left: w15 -> [w600]
    stop <- w597 stop-if-true
    # "Controller 1 - Mozgásérzékelõk adatai alapjánti beavatkozás a környezetbe."
    n287 = case shown="\"Update\"" w596 {
      tunnel: w601 -> [_ w628 _]
      tunnel: w600 -> [w606 w627 w693]
      tunnel: [w606 w611 w693] -> w599
      tunnel: [LightCases."Update" w623 LightCases."Stop"] -> w598
      tunnel: [FALSE FALSE TRUE] -> w597
      tunnel: w595 -> [w603 w619 w694]
      tunnel: [w603 w618 w694] -> w594
      frame "Start", Default {
        w602 = FALSE
        # "Lámpák"
        "B Lámpa" <- w602
        "N Lámpa" <- w602
        "FF Lámpa" <- w602
        "FM Lámpa" <- w602
        "KÉ Lámpa" <- w602
        "HSZ2 Lámpa" <- w602
        "HSZ1 Lámpa" <- w602
        "EF Lámpa" <- w602
        "LH Lámpa" <- w602
        "EM Lámpa" <- w602
        "RIASZTÁS" <- w602
      }
      frame "Update" {
        n288 = Dequeue Element(queue=w628, timeout in ms (-1)=100, error in (no error)=w627) -> (element=w621:T8, timed out?=w620:bool, error out=w608:errorcluster)  [unwired: 1 out]
        n289 = Select(t=w619, s=w620, f=w621) -> (s? t:f=w618:T8)
        n290 = call "LightOn FVG.vi"("Mode"=FVGFuncts."Get Data", "Error In"=w608) -> ("Error Out"=w609:errorcluster, "Data Out"=w610:bool)  [unwired: 8 in]
        n291 = case shown="True" w610 {
          tunnel: w618 -> [_ w642]
          tunnel: [w639 w641] -> w612
          tunnel: w609 -> [w639 w641]
          frame False {
            w640 = FALSE
            n292 = local write "HSZ2 Lámpa"(w640) -> ()
            n293 = local write "HSZ1 Lámpa"(w640) -> ()
            n294 = local write "B Lámpa"(w640) -> ()
            n295 = local write "N Lámpa"(w640) -> ()
            n296 = local write "FF Lámpa"(w640) -> ()
            n297 = local write "EF Lámpa"(w640) -> ()
            n298 = local write "FM Lámpa"(w640) -> ()
            n299 = local write "LH Lámpa"(w640) -> ()
            n300 = local write "EM Lámpa"(w640) -> ()
            n301 = local write "KÉ Lámpa"(w640) -> ()
          }
          frame True {
            n302 = for {
              N: 6 -> [_]
              tunnel: [w677] -> w648
              tunnel: w642 -> [w675] mode=indexing
              stop <- w677 stop-if-true
              n303 = Equal?(x=w675, y=Rooms."Lépcsõ" ("Enum")) -> (x = y?=w677:bool)
            }
            n304 = for {
              N: 6 -> [_]
              tunnel: [w692] -> w656
              tunnel: w642 -> [w690] mode=indexing
              stop <- w692 stop-if-true
              n305 = Equal?(x=w690, y=Rooms."Elõszoba" ("Enum")) -> (x = y?=w692:bool)
            }
            n306 = for {
              N: 6 -> [_]
              tunnel: [w686] -> w657
              tunnel: w642 -> [w684] mode=indexing
              stop <- w686 stop-if-true
              n307 = Equal?(x=w684, y=Rooms."Nappali" ("Enum")) -> (x = y?=w686:bool)
            }
            n308 = for {
              N: 6 -> [_]
              tunnel: [w674] -> w646
              tunnel: w642 -> [w672] mode=indexing
              stop <- w674 stop-if-true
              n309 = Equal?(x=w672, y=Rooms."Emeleti folyosó" ("Enum")) -> (x = y?=w674:bool)
            }
            n310 = for {
              N: 6 -> [_]
              tunnel: [w683] -> w654
              tunnel: w642 -> [w681] mode=indexing
              stop <- w683 stop-if-true
              n311 = Equal?(x=w681, y=Rooms."Földszinti mosdó" ("Enum")) -> (x = y?=w683:bool)
            }
            n312 = for {
              N: 6 -> [_]
              tunnel: [w680] -> w653
              tunnel: w642 -> [w678] mode=indexing
              stop <- w680 stop-if-true
              n313 = Equal?(x=w678, y=Rooms."Konyha" ("Enum")) -> (x = y?=w680:bool)
            }
            n314 = for {
              N: 6 -> [_]
              tunnel: [w671] -> w647
              tunnel: w642 -> [w669] mode=indexing
              stop <- w671 stop-if-true
              n315 = Equal?(x=w669, y=Rooms."Emeleti mosdó" ("Enum")) -> (x = y?=w671:bool)
            }
            n316 = for {
              N: 6 -> [_]
              tunnel: [w668] -> w644
              tunnel: w642 -> [w666] mode=indexing
              stop <- w668 stop-if-true
              n317 = Equal?(x=w666, y=Rooms."Hálószoba 1" ("Enum")) -> (x = y?=w668:bool)
            }
            n318 = for {
              N: 6 -> [_]
              tunnel: [w689] -> w655
              tunnel: w642 -> [w687] mode=indexing
              stop <- w689 stop-if-true
              n319 = Equal?(x=w687, y=Rooms."Földszinti folyosó" ("Enum")) -> (x = y?=w689:bool)
            }
            n320 = for {
              N: 6 -> [_]
              tunnel: [w665] -> w643
              tunnel: w642 -> [w663] mode=indexing
              stop <- w665 stop-if-true
              n321 = Equal?(x=w663, y=Rooms."Hálószoba 2" ("Enum")) -> (x = y?=w665:bool)
            }
            n322 = local write "HSZ2 Lámpa"(w643) -> ()
            n323 = local write "HSZ1 Lámpa"(w644) -> ()
            n324 = local write "B Lámpa"(w656) -> ()
            n325 = local write "N Lámpa"(w657) -> ()
            n326 = local write "FF Lámpa"(w655) -> ()
            n327 = local write "EF Lámpa"(w646) -> ()
            n328 = local write "FM Lámpa"(w654) -> ()
            n329 = local write "LH Lámpa"(w648) -> ()
            n330 = local write "EM Lámpa"(w647) -> ()
            n331 = local write "KÉ Lámpa"(w653) -> ()
          }
        }
        n332 = call "AlarmOn FVG.vi"("Mode"=FVGFuncts."Get Data", "Error In"=w608) -> ("Error Out"=w614:errorcluster, "Data Out"=w616:bool)  [unwired: 8 in]
        n333 = case shown="True" w616 {
          tunnel: w618 -> [_ w635]
          tunnel: [FALSE w633] -> w617
          tunnel: w614 -> [w630 w632]
          tunnel: [w630 w632] -> w613
          frame False {
          }
          frame True {
            n334 = for {
              N: 6 -> [_]
              tunnel: [w638] -> w633
              tunnel: w635 -> [w636] mode=indexing
              stop <- w638 stop-if-true
              n335 = Not Equal?(x=w636, y=Rooms."Sehol" ("Enum")) -> (x != y?=w638:bool)
            }
          }
        }
        n336 = local read "Stopped"() -> (w625:bool)
        n337 = local write "RIASZTÁS"(w617) -> ()
        n338 = Merge Errors(w608, w613, w612) -> (w611:errorcluster)
        n339 = Select(t=LightCases."Stop", s=w625, f=LightCases."Update") -> (s? t:f=w623:T4)
      }
      frame "Stop" {
      }
    }
    n340 = Wait Until Next ms Multiple(millisecond multiple=u32 200) -> ()  [unwired: 1 out]
  }
  n341 = Divide(x=1.0, y=w29) -> (x/y=w19:dbl)
  n342 = control-ref of="Stopped"() -> (w17:refnum<vi>)
  n343 = while {
    tunnel: w9 -> [w712]
    tunnel: w8 -> [w711]
    shift-right: [w709] -> _
    shift-left: LightCases."Start" -> [w713]
    shift-right: [w707] -> _
    shift-left: _ -> [w705]
    shift-right: [w708] -> _
    shift-left: _ -> [w706]
    shift-right: [w697] -> w2
    shift-left: w15 -> [w714]
    shift-right: [w703] -> _
    shift-left: w3 -> [w702]
    shift-right: [w704] -> _
    shift-left: w3 -> [w701]
    tunnel: w5 -> [w700]
    shift-right: [w699] -> _
    shift-left: _ -> [w698]
    stop <- w710 stop-if-true
    # "Modell - Set by INI file"
    n344 = case shown="\"Update\"" w713 {
      tunnel: w714 -> [w722 w789 w846]
      tunnel: w712 -> [w730 _ _]
      tunnel: w711 -> [w731 _ _]
      tunnel: [FALSE FALSE TRUE] -> w710
      tunnel: [LightCases."Update" w806 LightCases."Stop"] -> w709
      tunnel: [w721 w764 w845] -> w708
      tunnel: [w723 w765 w847] -> w707
      tunnel: [w722 w760 w846] -> w697
      tunnel: w706 -> [_ w764 w845]
      tunnel: w705 -> [_ w765 w847]
      tunnel: [w715 w775 w844] -> w704
      tunnel: [w716 w774 w843] -> w703
      tunnel: w702 -> [w716 w757 w843]
      tunnel: w701 -> [w715 w756 w844]
      tunnel: w700 -> [w718 _ _]
      tunnel: [w717 w735 w842] -> w699
      tunnel: w698 -> [_ w735 w842]
      frame "Start", Default {
        n345 = call-poly <vilib>:"Read From Spreadsheet File.vi"("file path (dialog if empty)"=w718) -> ("all rows"=w719:string[][])  [unwired: 6 in, 4 out]
        n346 = call-poly <vilib>:"Read From Spreadsheet File.vi"("file path (dialog if empty)"=w731) -> ("all rows"=w724:string[][])  [unwired: 6 in, 4 out]
        n347 = call-poly <vilib>:"Read From Spreadsheet File.vi"("file path (dialog if empty)"=w730) -> ("all rows"=w727:string[][])  [unwired: 6 in, 4 out]
        n348 = Delete From Array(array=w719, index (row)=0) -> (array with subset deleted=w717:string[][])  [unwired: 2 in, 1 out]
        n349 = Delete From Array(array=w727, index (row)=0) -> (array with subset deleted=w723:string[][])  [unwired: 2 in, 1 out]
        n350 = Delete From Array(array=w724, index (row)=0) -> (array with subset deleted=w721:string[][])  [unwired: 2 in, 1 out]
      }
      frame "Update" {
        w746 = "%d.%d" ("regular expression")
        w747 = 1 ("index (row)")
        w787 = "%d.%d" ("regular expression")
        n351 = Array Size(array=w764) -> (size(s)=w805:i32[])
        n352 = Array Size(array=w765) -> (size(s)=w800:i32[])
        n353 = Index Array(array=w805, index=0) -> (element=w803:i32)
        n354 = Index Array(array=w800, index=0) -> (element=w798:i32)
        n355 = Index Array(array=w735, index (row) #1=0 ("index (row)"), index (col) #1=w747, index (row) #2=w747, index (col) #2=w747) -> (element #1=w748:string, element #2=w745:string)
        n356 = Quotient & Remainder(x=w757, y=w803) -> (x-y*floor(x/y)=w802:i32)  [unwired: 1 out]
        n357 = Quotient & Remainder(x=w756, y=w798) -> (x-y*floor(x/y)=w797:i32)  [unwired: 1 out]
        n358 = Equal To 0?(x=w802) -> (x = 0?=w801:bool)
        n359 = Equal To 0?(x=w797) -> (x = 0?=w795:bool)
        n360 = call "Clock FVG.vi"("Mode"=FVGFuncts."Get Data", "Error In"=w789) -> ("Error Out"=w786:errorcluster, "Data Out"=w790:dbl)  [unwired: 8 in]
        n361 = Select(t=0 ("index"), s=w801, f=w757) -> (s? t:f=w758:i32)
        n362 = Select(t=0 ("index"), s=w795, f=w756) -> (s? t:f=w759:i32)
        n363 = Scan From String(format string=w746, input string=w748) -> (output 1=w739:i32, output 2=w740:i32)  [unwired: 4 in, 3 out]
        n364 = Index Array(array=w764, index (row)=w758) -> (element=w769:string[])  [unwired: 1 in]
        n365 = Index Array(array=w765, index (row)=w759) -> (element=w768:string[])  [unwired: 1 in]
        n366 = Format Date/Time String(time format string (%c)="%H.%M", seconds (now)=w790, UTC format=TRUE) -> (date/time string=w788:string)
        n367 = Scan From String(format string=w746, input string=w745) -> (output 1=w738:i32, output 2=w737:i32)  [unwired: 4 in, 3 out]
        n368 = Index Array(array=w769, index=0) -> (element=w771:string)
        n369 = Index Array(array=w768, index=0) -> (element=w770:string)
        n370 = Scan From String(format string=w787, input string=w788, error in=w786) -> (error out=w763:errorcluster, output 1=w751:i32, output 2=w736:i32)  [unwired: 3 in, 2 out]
        n371 = Scan From String(format string=w787, input string=w770, error in=w786) -> (error out=w766:errorcluster, output 1=w785:i32, output 2=w783:i32)  [unwired: 3 in, 2 out]
        n372 = Scan From String(format string=w787, input string=w771, error in=w786) -> (error out=w767:errorcluster, output 1=w784:i32, output 2=w782:i32)  [unwired: 3 in, 2 out]
        n373 = Equal?(x=w783, y=w736) -> (x = y?=w780:bool)
        n374 = Equal?(x=w782, y=w736) -> (x = y?=w778:bool)
        n375 = Equal?(x=w736, y=w740) -> (x = y?=w744:bool)
        n376 = Equal?(x=w751, y=w785) -> (x = y?=w781:bool)
        n377 = Equal?(x=w751, y=w784) -> (x = y?=w779:bool)
        n378 = Equal?(x=w736, y=w737) -> (x = y?=w741:bool)
        n379 = Equal?(x=w751, y=w738) -> (x = y?=w742:bool)
        n380 = And(x=w781, y=w780) -> (x .and. y?=w776:bool)
        n381 = And(x=w779, y=w778) -> (x .and. y?=w777:bool)
        n382 = case shown="True" w776 {
          tunnel: [w831 w841] -> w775
          tunnel: w759 -> [w831 w840]
          tunnel: w768 -> [_ w838]
          tunnel: w766 -> [w830 w834]
          tunnel: [w830 w832] -> w762
          frame False {
          }
          frame True {
            n383 = Index Array(array=w838, index=1) -> (element=w836:string)
            n384 = Equal?(x=w836, y="On") -> (x = y?=w833:bool)
            n385 = local write "Riasztó"(w833) -> ()
            n386 = call "AlarmOn FVG.vi"("Mode"=FVGFuncts."Set Data", "Error In"=w834, "Data In"=w833) -> ("Error Out"=w832:errorcluster)  [unwired: 7 in, 1 out]
            n387 = Increment(x=w840) -> (x+1=w841:i32)
          }
        }
        n388 = case shown="True" w777 {
          tunnel: w758 -> [w820 w829]
          tunnel: [w820 w828] -> w774
          tunnel: w769 -> [_ w827]
          tunnel: w767 -> [w818 w821]
          tunnel: [w816 w822] -> w761
          frame False {
            n389 = call "AlarmOn FVG.vi"("Mode"=FVGFuncts."Set Data", "Error In"=w818, "Data In"="Riasztó") -> ("Error Out"=w816:errorcluster)  [unwired: 7 in, 1 out]
          }
          frame True {
            n390 = Index Array(array=w827, index=1) -> (element=w824:string)
            n391 = Scan From String(format string="%f", input string=w824, error in=w821) -> (error out=w822:errorcluster, output 1=w823:dbl)  [unwired: 2 in, 2 out]
            n392 = local write "Kívánt hõm. F0"(w823) -> ()
            n393 = local write "Kívánt hõm. F1"(w823) -> ()
            n394 = Increment(x=w829) -> (x+1=w828:i32)
          }
        }
        n395 = Equal?(x=w751, y=w739) -> (x = y?=w750:bool)
        n396 = And(x=w750, y=w744) -> (x .and. y?=w743:bool)
        n397 = And(x=w742, y=w741) -> (x .and. y?=w734:bool)
        n398 = case shown="False" w743 {
          tunnel: w734 -> [w812 _]
          tunnel: [w811 w815] -> w732
          frame False {
            n399 = case shown="True" w812 {
              tunnel: ["Világítás" w814] -> w811
              frame False {
              }
              frame True {
                w814 = FALSE
                n400 = local write "Világítás"(w814) -> ()
              }
            }
          }
          frame True {
            w815 = TRUE
            n401 = local write "Világítás"(w815) -> ()
          }
        }
        n402 = call "LightOn FVG.vi"("Mode"=FVGFuncts."Set Data", "Data In"=w732) -> ()  [unwired: 8 in, 2 out]
        n403 = Wait Until Next ms Multiple(millisecond multiple=u32 200) -> ()  [unwired: 1 out]
        n404 = local read "Stopped"() -> (w807:bool)
        n405 = Select(t=LightCases."Start", s="Update Settings", f=LightCases."Update") -> (s? t:f=w752:T4)
        n406 = Merge Errors(w763, w762, w761) -> (w760:errorcluster)
        n407 = Select(t=LightCases."Stop", s=w807, f=w752) -> (s? t:f=w806:T4)
      }
      frame "Stop" {
      }
    }
  }
  n408 = while {
    tunnel: w7 -> [w850]
    shift-right: [w868] -> w16
    shift-left: w20 -> [w861]
    shift-right: [w863] -> _
    shift-left: LightCases."Start" -> [w864]
    shift-right: [w865] -> _
    shift-left: w22 -> [w866]
    tunnel: w19 -> [w854]
    shift-right: [w852] -> _
    shift-left: w21 -> [w853]
    tunnel: w17 -> [w855]
    i -> [w873]
    stop <- w851 stop-if-true
    # "Controller 2 - A környezeti adatok szimulált értékeinek beolvasása, majd ez alapjánti hõmérségletszimuláció a környezetben."
    n409 = call "TempSim SubVI.vi"("Stopped Boolean"=w855, "Temperature Queue in"=w850, "Frequency"=w854, "error in (no error)"=w861, "LightCases in"=w864, "Temperatures in"=w853, "TemperatureData in"=w866) -> ("TemperatureData out"=w865:T7, "Stop loop?"=w851:bool, "LightCases out"=w863:T4, "Temperatures out"=w852:T6, "F0 Temp Chart"=→"F0 Temp Chart":dbl, "F0 Gain"=→"F0 Gain":dbl, "Kinti hõmérséklet"=→"Kinti hõmérséklet":dbl, "F1 Temp Chart"=→"F1 Temp Chart":dbl, "F1 Gain"=→"F1 Gain":dbl, "error out"=w862:errorcluster)  [unwired: 3 in]
    n410 = Quotient & Remainder(x=w873, y=5.0) -> (x-y*floor(x/y)=w869:dbl, floor(x/y)=w871:dbl)
    n411 = Equal To 0?(x=w869) -> (x = 0?=w870:bool)
    n412 = case shown="True" w870 {
      tunnel: w871 -> [_ w879]
      tunnel: w861 -> [w874 w876]
      tunnel: [w874 w875] -> w867
      frame False {
      }
      frame True {
        n413 = Multiply(x=w879, y=60.0) -> (x*y=w877:dbl)
        n414 = call "Clock FVG.vi"("Mode"=FVGFuncts."Set Data", "Error In"=w876, "Data In"=w877) -> ("Error Out"=w875:errorcluster)  [unwired: 7 in, 1 out]
      }
    }
    n415 = Merge Errors(w862, w867) -> (w868:errorcluster)
  }
  n416 = Merge Errors(w24, w38, w16, w2) -> (w40:errorcluster)
  n417 = Release Queue(queue=w39, error in (no error)=w40) -> (error out=w26:errorcluster)  [unwired: 1 in, 2 out]
  n418 = Release Queue(queue=w7, error in (no error)=w26) -> (error out=w25:errorcluster)  [unwired: 1 in, 2 out]
  n419 = call <vilib>:"Simple Error Handler.vi"("error in (no error)"=w25) -> ("error out"=w1:errorcluster)  [unwired: 4 in, 4 out]
  n420 = call <vilib>:"Clear Errors.vi"("error in (no error)"=w1) -> ()  [unwired: 5 in, 2 out]
  n421 = disable-structure shown="Disabled" {
    frame Disabled {
      (unwired) Rooms."Sehol" ("element")
      n422 = xnode "Error Ring"() -> ()  [unwired: 1 out]
      n423 = Merge Errors() -> ()  [unwired: 3 in, 1 out]
      n424 = local read "Previous Button"() -> ()  [unwired: 1 out]
      n425 = local read "Previous Button"() -> (w883:bool)
      n426 = local read "Previous Button"() -> (w889:bool)
      n427 = local read "Next Button"() -> (w881:bool)
      n428 = local read "Down Button"() -> (w888:bool)
      n429 = local read "Next Button"() -> (w890:bool)
      n430 = local read "Up Button"() -> (w887:bool)
      n431 = local read "Down Button"() -> ()  [unwired: 1 out]
      n432 = local read "Up Button"() -> ()  [unwired: 1 out]
      n433 = local read "Next Button"() -> ()  [unwired: 1 out]
      n434 = Select(t=Rooms."Elõszoba" ("element"), s=w881, f=Rooms."Nappali" ("element")) -> (s? t:f=w886:T9)
      n435 = Compound Arithmetic op=OR(w890, w889, w888, w887) -> ()  [unwired: 1 out]
      n436 = Select(t=Rooms."Földszinti folyosó" ("element"), s=w883, f=w886) -> ()  [unwired: 1 out]
    }
    frame Enabled {
    }
  }
